vi "数据编码.vi"(0 "table输入":string(combo), 5 "错误常量 2":errorcluster caption="错误输入", 9 "QN":string, 13 "MN":string, 14 "PW":string) -> (4 "错误常量":errorcluster caption="错误输出", 15 "通讯包字符串":string)   [LabVIEW 2016, in "数据传输系统.lvlib"]
panel:
  out "核查数据发送次数":i32
  out "小时数据发送次数":i32
  out "长度":i32
  in  "数据块":T1
  out "通讯包":T2={"包头（2）"="##", "数据段长度（4）"="", "数据段"="", "CRC校验"="", "包尾"=""}
  # "范例代码：\n\n##0101QN=20160801085857223;ST=32;CN=1062;PW=100000;MN=010000A8900016F000169DC0;Flag=5\n;CP=&&RtdInterval=30&&1C80\\r\\n"
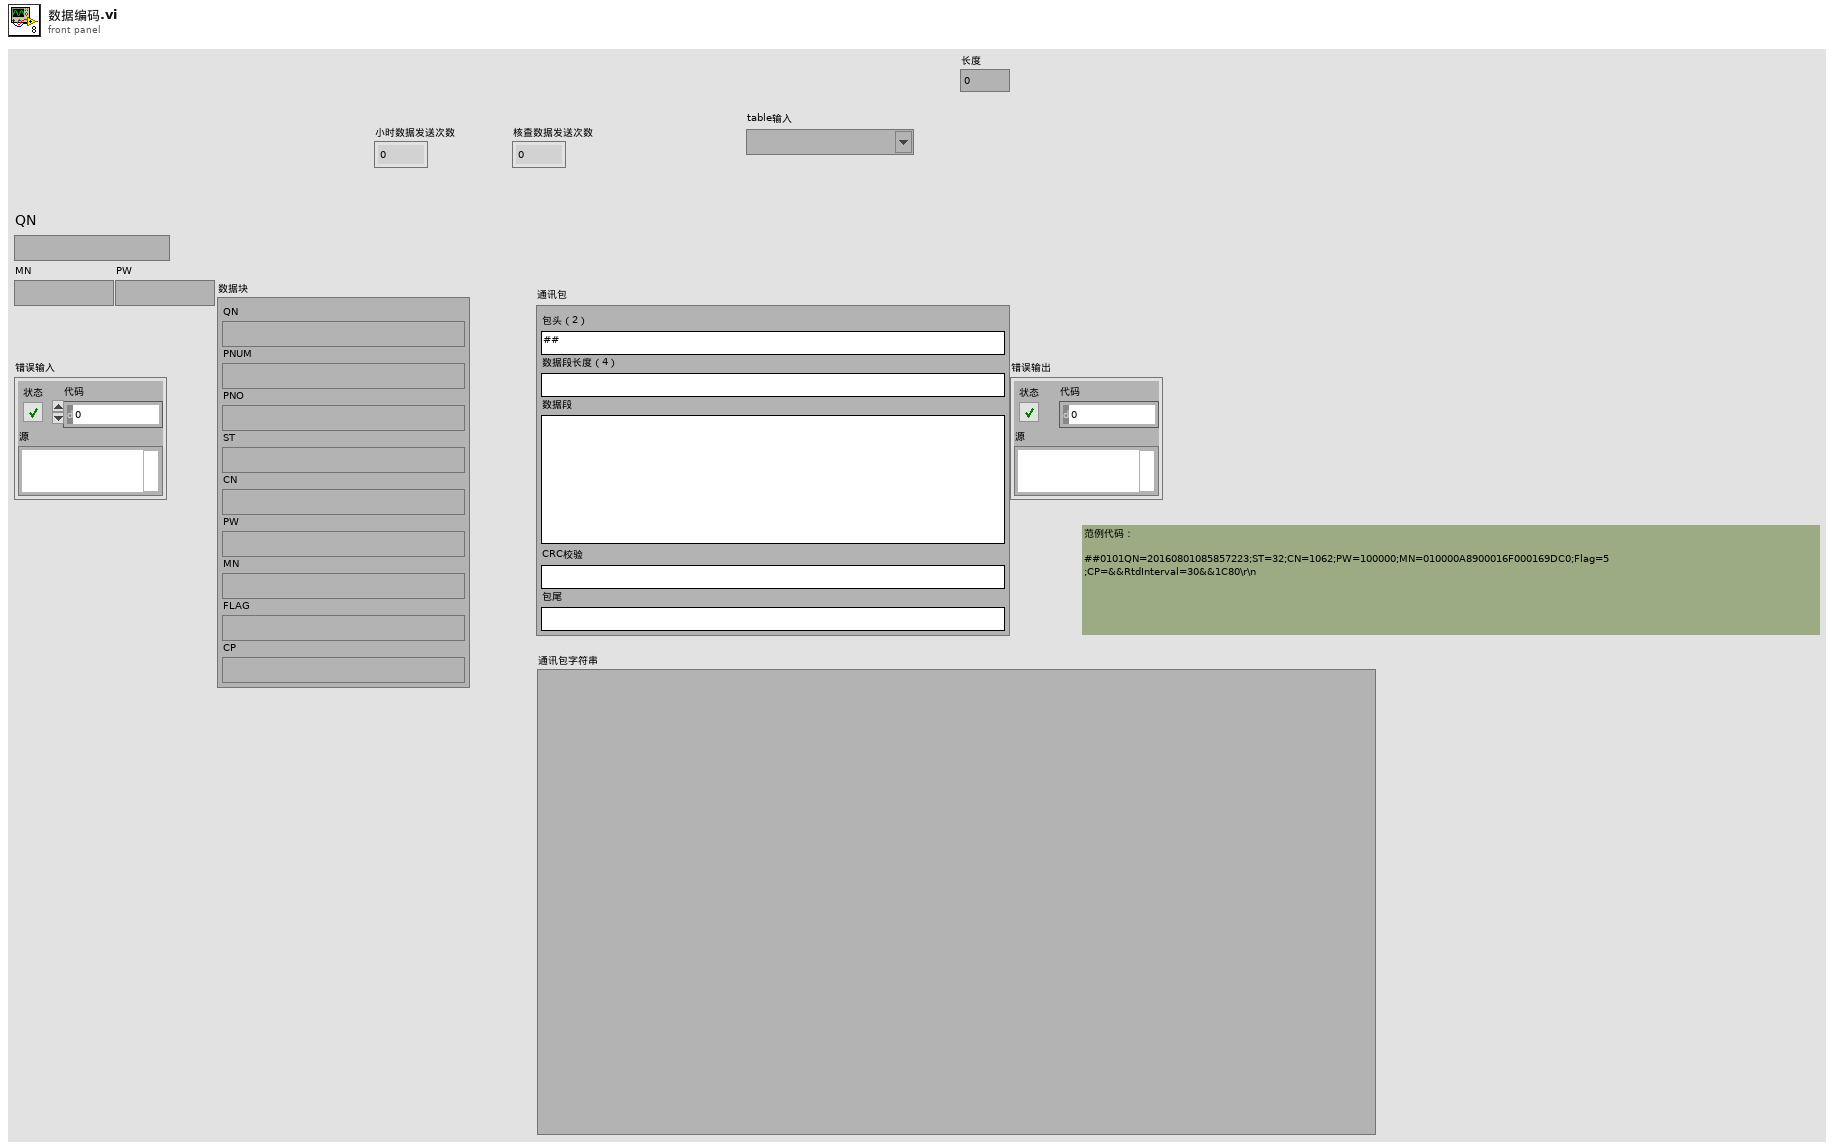
[diagram p1: front panel]
types:
  T1 = cluster{"QN":string, "ST":string, "CN":string, "PW":string, "MN":string, "FLAG":string, "PNUM":string, "PNO":string, "CP":string}
  T2 = cluster{"包头（2）":string, "数据段长度（4）":string, "数据段":string, "CRC校验":string, "包尾":string}
  T3 = cluster{"PH":string[][], "CODCr":string[][], "氨氮":string[][], "CODMn":string[][], "总氮":string[][], "总磷":string[][], "电导率":string[][], "水温":string[][], "DO":string[][], "浊度":string[][], "叶绿素":string[][], "藻密度":string[][], "铜":string[][], "盐度":string[][], "水位":string[][], "流速":string[][], "瞬时流量":string[][], "累积流量":string[][], "亚硝酸盐":string[][], "硫化物":string[][], "ORP":string[][], "铅":string[][], "镉":string[][], "锌":string[][], "镍":string[][], "锰":string[][], "汞":string[][], "气温":string[][], "气压":string[][], "风速":string[][], "风向":string[][]}
  T4 = enum16{"小时数据", "实时数据", "平行样测试", "集成干预测试", "加标回收测试", "核查数据", "空白零点跨度数据", "提取小时数据", "提取实时数据"}
  T5 = enum16{"小时数据", "实时数据", "平行样测试", "集成干预测试", "加标回收测试", "核查数据", "空白零点跨度数据", "提取小时数据", "提取实时数据", "操作日志"}
  T6 = enum16{"小时数据", "实时数据", "平行样测试", "集成干预测试", "加标回收测试", "核查数据", "空白零点跨度数据", "提取小时数据", "提取实时数据", "操作日志", "仪器参数", "3090仪器参数", "提取仪器参数", "报警信息"}
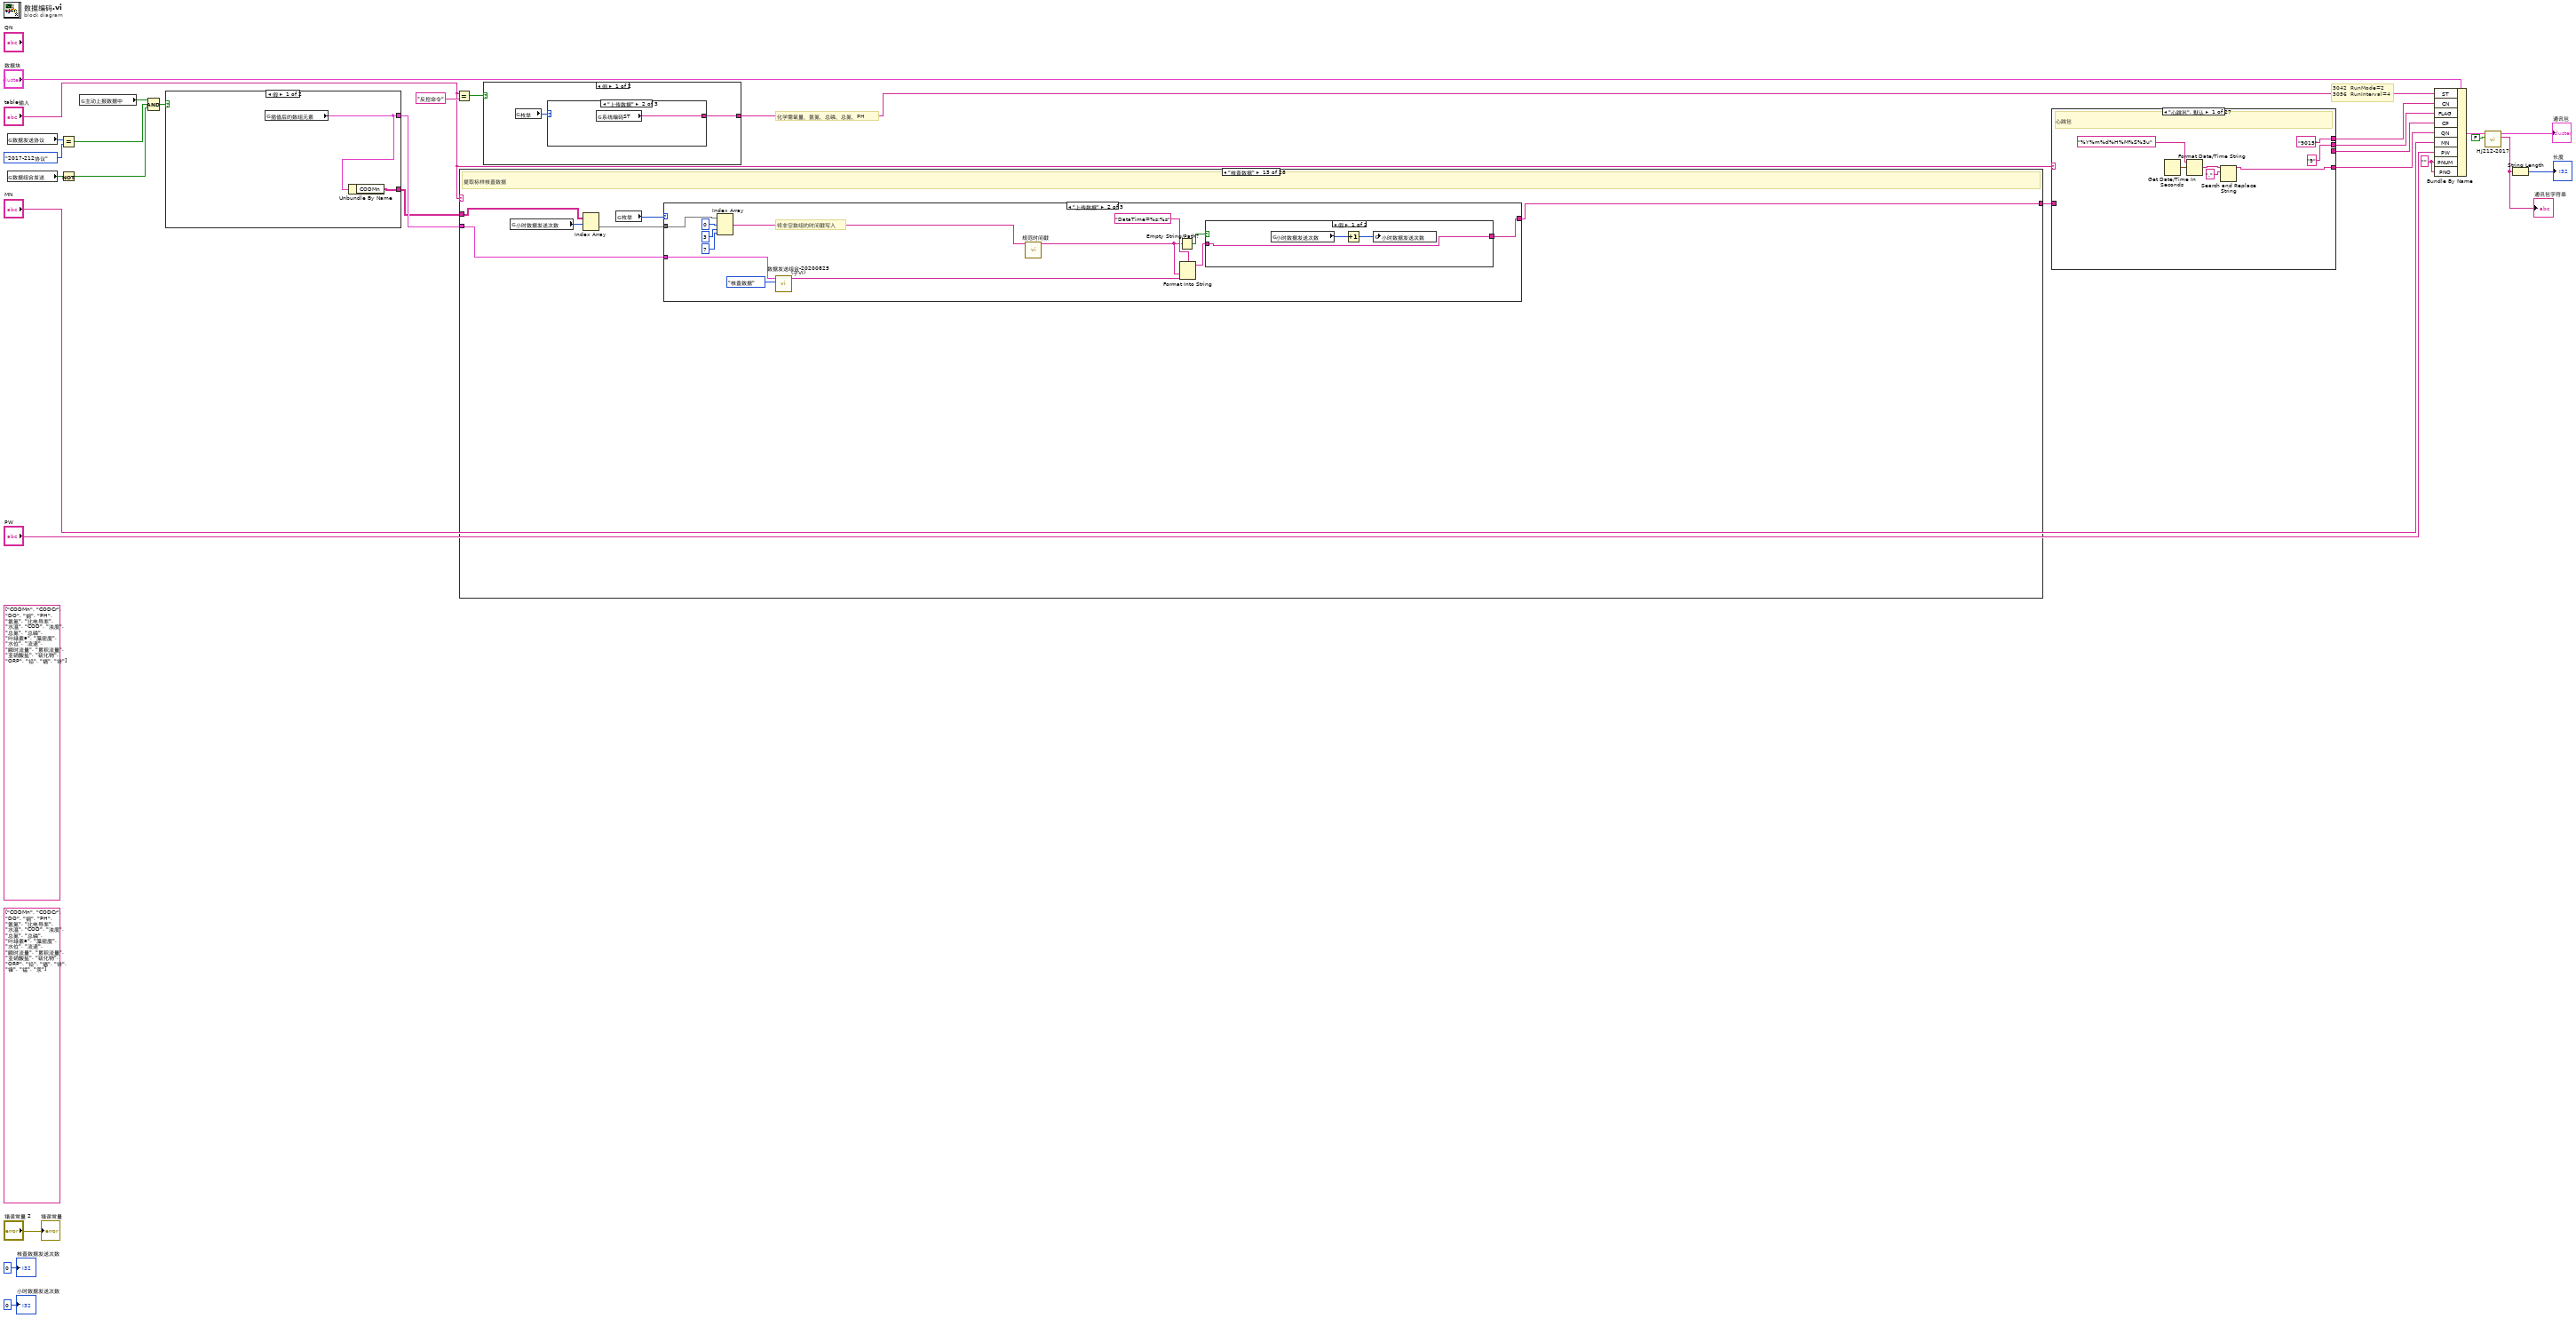
[diagram p0: block diagram]
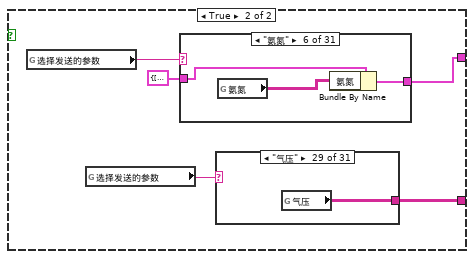
[diagram p2: hidden frame]
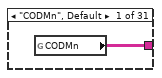
[diagram p3: hidden frame]
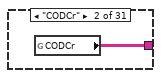
[diagram p4: hidden frame]
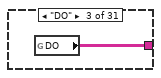
[diagram p5: hidden frame]
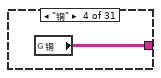
[diagram p6: hidden frame]
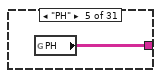
[diagram p7: hidden frame]
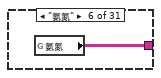
[diagram p8: hidden frame]
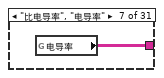
[diagram p9: hidden frame]
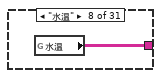
[diagram p10: hidden frame]
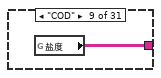
[diagram p11: hidden frame]
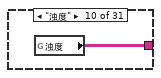
[diagram p12: hidden frame]
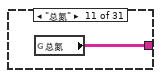
[diagram p13: hidden frame]
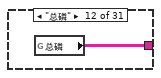
[diagram p14: hidden frame]
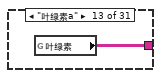
[diagram p15: hidden frame]
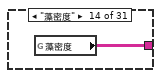
[diagram p16: hidden frame]
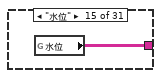
[diagram p17: hidden frame]
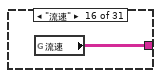
[diagram p18: hidden frame]
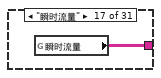
[diagram p19: hidden frame]
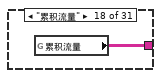
[diagram p20: hidden frame]
diagram:
  (unwired) string[] ["CODMn", "CODCr", "DO", "铜", "PH", "氨氮", "比电导率", "水温", "COD", "浊度", "总氮", "总磷", "叶绿素a", "藻密度", "水位", "流速", "瞬时流量", "累积流量", "亚硝酸盐", "硫化物", "ORP", "铅", "镉", "锌"] ("数组")
  (unwired) string[] ["CODMn", "CODCr", "DO", "铜", "PH", "氨氮", "比电导率", "水温", "COD", "浊度", "总氮", "总磷", "叶绿素a", "藻密度", "水位", "流速", "瞬时流量", "累积流量", "亚硝酸盐", "硫化物", "ORP", "铅", "镉", "锌", "镍", "锰", "汞"] ("数组")
  w15 = ""
  # "化学需氧量、氨氮、总磷、总氮、PH"
  # "3042  RunMode=2\n3056  RunInterval=4"
  n1 = global read "断电保存全局.vi" "数据发送协议"() -> (w5:enum16{"2005-212协议", "2017-212协议"})
  n2 = global read "断电保存全局.vi" "数据组合发送"() -> (w7:bool)
  n3 = Equal?(x=w5, y=enum16{"2005-212协议", "2017-212协议"}."2017-212协议" ("数据发送版本")) -> (x = y?=w8:bool)
  n4 = Not(x=w7) -> (.not. x?=w6:bool)
  n5 = global read "全局 数据发送重叠.vi" "主动上报数据中"() -> (w12:bool)
  n6 = Compound Arithmetic op=AND ("复合运算")(w12, w8, w6) -> (w9:bool)
  n7 = case shown="假" w9 {
    tunnel: [w32 w36] -> w3
    tunnel: [w31 w33] -> w1
    frame False {
      n8 = global read "插值后的新数组.vi" "插值后的数组元素"() -> (w32:T3)
      n9 = Unbundle By Name(w32) -> ("CODMn"=w31:string[][])
    }
    frame True {
      n10 = global read "全局 水样时间.vi" "选择发送的参数"() -> (w37:string)
      n11 = global read "全局 水样时间.vi" "选择发送的参数"() -> (w34:string)
      n12 = case shown="\"氨氮\"" w37 {
        tunnel: T3 {"PH"=[], "CODCr"=[], "氨氮"=[], "CODMn"=[], "总氮"=[], "总磷"=[], "电导率"=[], "水温"=[], "DO"=[], "浊度"=[], "叶绿素"=[], "藻密度"=[], "铜"=[], "盐度"=[], "水位"=[], "流速"=[], "瞬时流量"=[], "累积流量"=[], "亚硝酸盐"=[], "硫化物"=[], "ORP"=[], "铅"=[], "镉"=[], "锌"=[], "镍"=[], "锰"=[], "汞"=[], "气温"=[], "气压"=[], "风速"=[], "风向"=[]} ("插值后的数组元素") -> [w70 w74 w77 w80 w83 w86 w89 w92 w95 w98 w101 w104 w107 w109 w113 w116 w118 w121 w124 w127 w130 w133 w136 w139 w142 w145 w148 w151 w154 w157 w160]
        tunnel: [w69 w72 w75 w78 w81 w84 w88 w91 w93 w96 w99 w102 w105 w108 w111 w114 w117 w120 w123 w126 w129 w132 w135 w138 w141 w144 w147 w150 w153 w156 w159] -> w36
        frame "CODMn", Default {
          n13 = global read "全局 所有参数.vi" "CODMn"() -> (w71:string[][])
          n14 = Bundle By Name(cluster=w70, "CODMn"=w71) -> (w69:T3)
        }
        frame "CODCr" {
          n15 = global read "全局 所有参数.vi" "CODCr"() -> (w73:string[][])
          n16 = Bundle By Name(cluster=w74, "CODCr"=w73) -> (w72:T3)
        }
        frame "DO" {
          n17 = global read "全局 所有参数.vi" "DO"() -> (w76:string[][])
          n18 = Bundle By Name(cluster=w77, "DO"=w76) -> (w75:T3)
        }
        frame "铜" {
          n19 = global read "全局 所有参数.vi" "铜"() -> (w79:string[][])
          n20 = Bundle By Name(cluster=w80, "铜"=w79) -> (w78:T3)
        }
        frame "PH" {
          n21 = global read "全局 所有参数.vi" "PH"() -> (w82:string[][])
          n22 = Bundle By Name(cluster=w83, "PH"=w82) -> (w81:T3)
        }
        frame "氨氮" {
          n23 = global read "全局 所有参数.vi" "氨氮"() -> (w85:string[][])
          n24 = Bundle By Name(cluster=w86, "氨氮"=w85) -> (w84:T3)
        }
        frame "比电导率", "电导率" {
          n25 = global read "全局 所有参数.vi" "电导率"() -> (w87:string[][])
          n26 = Bundle By Name(cluster=w89, "电导率"=w87) -> (w88:T3)
        }
        frame "水温" {
          n27 = global read "全局 所有参数.vi" "水温"() -> (w90:string[][])
          n28 = Bundle By Name(cluster=w92, "水温"=w90) -> (w91:T3)
        }
        frame "COD" {
          n29 = global read "全局 所有参数.vi" "盐度"() -> (w94:string[][])
          n30 = Bundle By Name(cluster=w95, "盐度"=w94) -> (w93:T3)
        }
        frame "浊度" {
          n31 = global read "全局 所有参数.vi" "浊度"() -> (w97:string[][])
          n32 = Bundle By Name(cluster=w98, "浊度"=w97) -> (w96:T3)
        }
        frame "总氮" {
          n33 = global read "全局 所有参数.vi" "总氮"() -> (w100:string[][])
          n34 = Bundle By Name(cluster=w101, "总氮"=w100) -> (w99:T3)
        }
        frame "总磷" {
          n35 = global read "全局 所有参数.vi" "总磷"() -> (w103:string[][])
          n36 = Bundle By Name(cluster=w104, "总磷"=w103) -> (w102:T3)
        }
        frame "叶绿素a" {
          n37 = global read "全局 所有参数.vi" "叶绿素"() -> (w106:string[][])
          n38 = Bundle By Name(cluster=w107, "叶绿素"=w106) -> (w105:T3)
        }
        frame "藻密度" {
          n39 = global read "全局 所有参数.vi" "藻密度"() -> (w110:string[][])
          n40 = Bundle By Name(cluster=w109, "藻密度"=w110) -> (w108:T3)
        }
        frame "水位" {
          n41 = global read "全局 所有参数.vi" "水位"() -> (w112:string[][])
          n42 = Bundle By Name(cluster=w113, "水位"=w112) -> (w111:T3)
        }
        frame "流速" {
          n43 = global read "全局 所有参数.vi" "流速"() -> (w115:string[][])
          n44 = Bundle By Name(cluster=w116, "流速"=w115) -> (w114:T3)
        }
        frame "瞬时流量" {
          n45 = global read "全局 所有参数.vi" "瞬时流量"() -> (w119:string[][])
          n46 = Bundle By Name(cluster=w118, "瞬时流量"=w119) -> (w117:T3)
        }
        frame "累积流量" {
          n47 = global read "全局 所有参数.vi" "累积流量"() -> (w122:string[][])
          n48 = Bundle By Name(cluster=w121, "累积流量"=w122) -> (w120:T3)
        }
        frame "亚硝氮" {
          n49 = global read "全局 所有参数.vi" "亚硝酸盐"() -> (w125:string[][])
          n50 = Bundle By Name(cluster=w124, "亚硝酸盐"=w125) -> (w123:T3)
        }
        frame "硫化物" {
          n51 = global read "全局 所有参数.vi" "硫化物"() -> (w128:string[][])
          n52 = Bundle By Name(cluster=w127, "硫化物"=w128) -> (w126:T3)
        }
        frame "ORP" {
          n53 = global read "全局 所有参数.vi" "ORP"() -> (w131:string[][])
          n54 = Bundle By Name(cluster=w130, "ORP"=w131) -> (w129:T3)
        }
        frame "铅" {
          n55 = global read "全局 所有参数.vi" "铅"() -> (w134:string[][])
          n56 = Bundle By Name(cluster=w133, "铅"=w134) -> (w132:T3)
        }
        frame "镉" {
          n57 = global read "全局 所有参数.vi" "镉"() -> (w137:string[][])
          n58 = Bundle By Name(cluster=w136, "镉"=w137) -> (w135:T3)
        }
        frame "锌" {
          n59 = global read "全局 所有参数.vi" "锌"() -> (w140:string[][])
          n60 = Bundle By Name(cluster=w139, "锌"=w140) -> (w138:T3)
        }
        frame "镍" {
          n61 = global read "全局 所有参数.vi" "镍"() -> (w143:string[][])
          n62 = Bundle By Name(cluster=w142, "镍"=w143) -> (w141:T3)
        }
        frame "锰" {
          n63 = global read "全局 所有参数.vi" "锰"() -> (w146:string[][])
          n64 = Bundle By Name(cluster=w145, "锰"=w146) -> (w144:T3)
        }
        frame "汞" {
          n65 = global read "全局 所有参数.vi" "汞"() -> (w149:string[][])
          n66 = Bundle By Name(cluster=w148, "汞"=w149) -> (w147:T3)
        }
        frame "气温" {
          n67 = global read "全局 所有参数.vi" "气温"() -> (w152:string[][])
          n68 = Bundle By Name(cluster=w151, "气温"=w152) -> (w150:T3)
        }
        frame "气压" {
          n69 = global read "全局 所有参数.vi" "气压"() -> (w155:string[][])
          n70 = Bundle By Name(cluster=w154, "气压"=w155) -> (w153:T3)
        }
        frame "风速" {
          n71 = global read "全局 所有参数.vi" "风速"() -> (w158:string[][])
          n72 = Bundle By Name(cluster=w157, "风速"=w158) -> (w156:T3)
        }
        frame "风向" {
          n73 = global read "全局 所有参数.vi" "风向"() -> (w161:string[][])
          n74 = Bundle By Name(cluster=w160, "风向"=w161) -> (w159:T3)
        }
      }
      n75 = case shown="\"气压\"" w34 {
        tunnel: [w38 w39 w40 w41 w42 w43 w44 w45 w46 w47 w48 w49 w50 w51 w52 w53 w54 w55 w56 w57 w58 w59 w60 w61 w62 w63 w64 w65 w66 w67 w68] -> w33
        frame "CODMn", Default {
          n76 = global read "全局 所有参数.vi" "CODMn"() -> (w38:string[][])
        }
        frame "CODCr" {
          n77 = global read "全局 所有参数.vi" "CODCr"() -> (w39:string[][])
        }
        frame "DO" {
          n78 = global read "全局 所有参数.vi" "DO"() -> (w40:string[][])
        }
        frame "铜" {
          n79 = global read "全局 所有参数.vi" "铜"() -> (w41:string[][])
        }
        frame "PH" {
          n80 = global read "全局 所有参数.vi" "PH"() -> (w42:string[][])
        }
        frame "氨氮" {
          n81 = global read "全局 所有参数.vi" "氨氮"() -> (w43:string[][])
        }
        frame "比电导率", "电导率" {
          n82 = global read "全局 所有参数.vi" "电导率"() -> (w44:string[][])
        }
        frame "水温" {
          n83 = global read "全局 所有参数.vi" "水温"() -> (w45:string[][])
        }
        frame "COD" {
          n84 = global read "全局 所有参数.vi" "盐度"() -> (w46:string[][])
        }
        frame "浊度" {
          n85 = global read "全局 所有参数.vi" "浊度"() -> (w47:string[][])
        }
        frame "总氮" {
          n86 = global read "全局 所有参数.vi" "总氮"() -> (w48:string[][])
        }
        frame "总磷" {
          n87 = global read "全局 所有参数.vi" "总磷"() -> (w49:string[][])
        }
        frame "叶绿素a" {
          n88 = global read "全局 所有参数.vi" "叶绿素"() -> (w50:string[][])
        }
        frame "藻密度" {
          n89 = global read "全局 所有参数.vi" "藻密度"() -> (w51:string[][])
        }
        frame "水位" {
          n90 = global read "全局 所有参数.vi" "水位"() -> (w52:string[][])
        }
        frame "流速" {
          n91 = global read "全局 所有参数.vi" "流速"() -> (w53:string[][])
        }
        frame "瞬时流量" {
          n92 = global read "全局 所有参数.vi" "瞬时流量"() -> (w54:string[][])
        }
        frame "累积流量" {
          n93 = global read "全局 所有参数.vi" "累积流量"() -> (w55:string[][])
        }
        frame "亚硝氮" {
          n94 = global read "全局 所有参数.vi" "亚硝酸盐"() -> (w56:string[][])
        }
        frame "硫化物" {
          n95 = global read "全局 所有参数.vi" "硫化物"() -> (w57:string[][])
        }
        frame "ORP" {
          n96 = global read "全局 所有参数.vi" "ORP"() -> (w58:string[][])
        }
        frame "铅" {
          n97 = global read "全局 所有参数.vi" "铅"() -> (w59:string[][])
        }
        frame "镉" {
          n98 = global read "全局 所有参数.vi" "镉"() -> (w60:string[][])
        }
        frame "锌" {
          n99 = global read "全局 所有参数.vi" "锌"() -> (w61:string[][])
        }
        frame "镍" {
          n100 = global read "全局 所有参数.vi" "镍"() -> (w62:string[][])
        }
        frame "锰" {
          n101 = global read "全局 所有参数.vi" "锰"() -> (w63:string[][])
        }
        frame "汞" {
          n102 = global read "全局 所有参数.vi" "汞"() -> (w64:string[][])
        }
        frame "气温" {
          n103 = global read "全局 所有参数.vi" "气温"() -> (w65:string[][])
        }
        frame "气压" {
          n104 = global read "全局 所有参数.vi" "气压"() -> (w66:string[][])
        }
        frame "风速" {
          n105 = global read "全局 所有参数.vi" "风速"() -> (w67:string[][])
        }
        frame "风向" {
          n106 = global read "全局 所有参数.vi" "风向"() -> (w68:string[][])
        }
      }
    }
  }
  n107 = Equal?(x="table输入", y="反控命令") -> (x = y?=w19:bool)
  n108 = case shown="\"核查数据\"" "table输入" {
    tunnel: [w163 w170 w184 w227 w250 _ w264 w273 w284 w434 w465 w512 w563 w592 w624 w655 w681 w710 w739 w776 w810 w841 w869 w892 w925 w948 w959 w970] -> w13
    tunnel: w1 -> [_ _ _ _ _ _ _ _ w281 w433 _ _ w562 w593 w619 w650 w682 w709 w738 w775 w809 w840 _ w891 _ _ _ _]
    tunnel: w3 -> [_ _ _ _ _ _ _ _ w282 w435 _ _ w558 w588 w620 w651 w680 w708 w737 w771 w805 w836 w867 w887 _ _ _ _]
    frame "反控命令" {
      n109 = global read "全局 反控命令枚举.vi" "反控命令枚举"() -> (w162:enum16{"返回请求应答", "返回执行结果"})
      n110 = case shown="\"返回执行结果\"" w162 {
        tunnel: ["QnRtn=1" w166] -> w163
        frame "返回请求应答", Default {
        }
        frame "返回执行结果" {
          n111 = global read "全局 反控命令枚举.vi" "执行结果定义"() -> (w167:u16)
          n112 = Number To Decimal String(number=w167) -> (decimal integer string=w165:string)  [unwired: 1 in]
          n113 = Concatenate Strings("ExeRtn=", w165) -> (w166:string)
        }
      }
    }
    frame "超标留样返回" {
      n114 = global read "全局1.vi" "枚举"() -> (w169:enum16{"返回请求应答", "上传数据", "返回执行结果"})
      n115 = case shown="\"返回请求应答\", 默认" w169 {
        tunnel: ["QnRtn=1" w172 "ExeRtn=1"] -> w170
        frame "返回请求应答", Default {
        }
        frame "上传数据" {
          n116 = global read "全局1.vi" "register values"() -> (w181:u16[])
          n117 = Get Date/Time In Seconds() -> (seconds since 1Jan1904=w179:timestamp)
          n118 = Index Array(array=w181, index=7 ("索引")) -> (element=w174:u16)
          n119 = Format Date/Time String(time format string (%c)="%Y%m%d%H%M%S" ("时间格式字符串(%c)"), seconds (now)=w179) -> (date/time string=w177:string)  [unwired: 1 in]
          n120 = Number To Decimal String(number=w174) -> (decimal integer string=w175:string)  [unwired: 1 in]
          n121 = Format Into String(format string="VaseNo=%s" ("格式字符串"), w175) -> (resulting string=w173:string)  [unwired: 2 in, 1 out]
          n122 = Format Into String(format string="DataTime=%s;%s" ("格式字符串"), w177, w173) -> (resulting string=w172:string)  [unwired: 2 in, 1 out]
        }
        frame "返回执行结果" {
        }
      }
    }
    frame "提取经纬度环境信息" {
      # "BDS纬度"
      # "BDS纬度"
      # "GPS纬度"
      # "GPS经度"
      # "湿度"
      # "温度"
      # "电压"
      # "时间"
      n123 = global read "全局1.vi" "枚举"() -> (w185:enum16{"返回请求应答", "上传数据", "返回执行结果"})
      n124 = case shown="\"上传数据\"" w185 {
        tunnel: ["QnRtn=1" w198 "ExeRtn=1"] -> w184
        frame "返回请求应答", Default {
        }
        frame "上传数据" {
          n125 = global read "全局 环境参数.vi" "环境参数"() -> (w188:string[][])
          n126 = global read "全局 环境参数.vi" "columns输出"() -> (w195:string[])
          n127 = Index Array(array=w188, index (row)=0 ("索引 (行)")) -> (element=w191:string[])  [unwired: 1 in]
          n128 = Get Date/Time In Seconds() -> (seconds since 1Jan1904=w200:timestamp)
          n129 = Array Subset(array=w195, index=1 ("索引")) -> (w196:string[])  [unwired: 1 in]
          n130 = for {
            tunnel: w196 -> [w204] mode=indexing
            tunnel: [w203] -> w197 mode=indexing
            n131 = case shown="\"BDS经度\"" w204 {
              tunnel: ["" "Volt=%s;" "Temp=%s;" ("格式字符串") "Hum=%s;" ("格式字符串") "Lng=%s;" "Lat=%s;" "Lng2=%s;" "Lat2=%s;"] -> w203
              frame "假", Default {
              }
              frame "电压" {
              }
              frame "室温" {
              }
              frame "湿度" {
              }
              frame "GPS经度" {
              }
              frame "GPS纬度" {
              }
              frame "BDS经度" {
              }
              frame "BDS纬度" {
              }
            }
          }
          n132 = Format Date/Time String(time format string (%c)="%Y%m%d%H%M%S" ("时间格式字符串(%c)"), seconds (now)=w200) -> (date/time string=w199:string)  [unwired: 1 in]
          n133 = Array Subset(array=w191, index=1 ("索引")) -> (w193:string[])  [unwired: 1 in]
          n134 = for {
            shift-right: [w218] -> w187
            shift-left: "" -> [w217]
            tunnel: w197 -> [w216] mode=indexing
            tunnel: w193 -> [w214] mode=indexing
            n135 = Empty String/Path?(string/path=w214) -> (empty?=w220:bool)
            n136 = Fract/Exp String To Number(string=w214) -> (number=w215:dbl)  [unwired: 3 in, 1 out]
            n137 = Number To Fractional String(number=w215) -> (F-format string=w213:string)  [unwired: 3 in]
            n138 = case shown="假" w220 {
              tunnel: [w223 w224] -> w219
              tunnel: w216 -> [w222 _]
              tunnel: w213 -> [w221 _]
              tunnel: w213 -> [_ w224]
              frame False {
                n139 = Format Into String(format string=w222, w221) -> (resulting string=w223:string)  [unwired: 2 in, 1 out]
              }
              frame True {
              }
            }
            n140 = Concatenate Strings(w217, w219) -> (w218:string)
          }
          n141 = Format Into String(format string="DataTime=%s;%s" ("格式字符串"), w199, w187) -> (resulting string=w198:string)  [unwired: 2 in, 1 out]
        }
        frame "返回执行结果" {
        }
      }
    }
    frame "提取现场系统信息" {
      n142 = global read "全局1.vi" "枚举"() -> (w226:enum16{"返回请求应答", "上传数据", "返回执行结果"})
      n143 = case shown="\"上传数据\"" w226 {
        tunnel: ["QnRtn=1" w247 "ExeRtn=1"] -> w227
        frame "返回请求应答", Default {
        }
        frame "上传数据" {
          n144 = global read "全局1.vi" "register values"() -> (w246:u16[])
          n145 = Index Array(array=w246, index #1=0 ("索引"), index #2=6 ("索引")) -> (element #1=w242:u16, element #2=w229:u16)
          n146 = Number To Decimal String(number=w242) -> (decimal integer string=w244:string)  [unwired: 1 in]
          n147 = Number To Decimal String(number=w229) -> (decimal integer string=w238:string)  [unwired: 1 in]
          n148 = Get Date/Time In Seconds() -> (seconds since 1Jan1904=w232:timestamp)
          n149 = Format Date/Time String(time format string (%c)="%Y%m%d%H%M%S%u" ("时间格式字符串(%c)"), seconds (now)=w232) -> (date/time string=w235:string)  [unwired: 1 in]
          n150 = Format Into String(format string="RunMode=%s;" ("格式字符串"), w244) -> (resulting string=w241:string)  [unwired: 2 in, 1 out]
          n151 = Format Into String(format string="RunInterval=%s;" ("格式字符串"), w238) -> (resulting string=w239:string)  [unwired: 2 in, 1 out]
          n152 = Search and Replace String(input string=w235, search string="." ("搜索字符串")) -> (result string=w231:string)  [unwired: 6 in, 3 out]
          n153 = Format Into String(format string="SystemTime=%s;" ("格式字符串"), w231) -> (resulting string=w236:string)  [unwired: 2 in, 1 out]
          n154 = Concatenate Strings(w241, w239, w236) -> (w247:string)
        }
        frame "返回执行结果" {
        }
      }
    }
    frame "提取监测仪表时间" {
      n155 = global read "全局1.vi" "枚举"() -> (w249:enum16{"返回请求应答", "上传数据", "返回执行结果"})
      n156 = case shown="\"上传数据\"" w249 {
        tunnel: ["QnRtn=1" w262 "ExeRtn=1"] -> w250
        frame "返回请求应答", Default {
        }
        frame "上传数据" {
          n157 = global read "全局 提取仪器参数.vi" "仪器编码"() -> (w252:string)
          n158 = Format Into String(format string="PolId=%s;" ("格式字符串"), w252) -> (resulting string=w260:string)  [unwired: 2 in, 1 out]
          n159 = Get Date/Time In Seconds() -> (seconds since 1Jan1904=w255:timestamp)
          n160 = Format Date/Time String(time format string (%c)="%Y%m%d%H%M%S%u" ("时间格式字符串(%c)"), seconds (now)=w255) -> (date/time string=w258:string)  [unwired: 1 in]
          n161 = Search and Replace String(input string=w258, search string="." ("搜索字符串")) -> (result string=w254:string)  [unwired: 6 in, 3 out]
          n162 = Format Into String(format string="SystemTime=%s;" ("格式字符串"), w254) -> (resulting string=w253:string)  [unwired: 2 in, 1 out]
          n163 = Concatenate Strings(w260, w253) -> (w262:string)
        }
        frame "返回执行结果" {
        }
      }
    }
    frame "心跳包", Default {
    }
    frame "提取数采仪时间" {
      (unwired) ""
      n164 = global read "全局1.vi" "枚举"() -> (w265:enum16{"返回请求应答", "上传数据", "返回执行结果"})
      n165 = case shown="\"上传数据\"" w265 {
        tunnel: ["QnRtn=1" w267 "ExeRtn=1"] -> w264
        frame "返回请求应答", Default {
        }
        frame "上传数据" {
          n166 = Get Date/Time In Seconds() -> (seconds since 1Jan1904=w271:timestamp)
          n167 = Format Date/Time String(time format string (%c)="%Y%m%d%H%M%S" ("时间格式字符串(%c)"), seconds (now)=w271) -> (date/time string=w268:string)  [unwired: 1 in]
          n168 = Concatenate Strings("SystemTime=", w268) -> (w267:string)
        }
        frame "返回执行结果" {
        }
      }
    }
    frame "提取实时数据间隔" {
      (unwired) ""
      n169 = global read "全局1.vi" "枚举"() -> (w274:enum16{"返回请求应答", "上传数据", "返回执行结果"})
      n170 = case shown="\"上传数据\"" w274 {
        tunnel: ["QnRtn=1" w278 "ExeRtn=1"] -> w273
        frame "返回请求应答", Default {
        }
        frame "上传数据" {
          n171 = global read "实时数据发送间隔全局.vi" "实时数据发送间隔"() -> (w277:u32)
          n172 = Number To Decimal String(number=w277) -> (decimal integer string=w276:string)  [unwired: 1 in]
          n173 = Concatenate Strings("RtdInterval=", w276) -> (w278:string)
        }
        frame "返回执行结果" {
        }
      }
    }
    frame "实时数据" {
      # "包含质控数据主动上传"
      n174 = global read "全局 实时数据参数.vi" "实时数据参数"() -> (w283:string)
      n175 = case shown="\"水样测试\", 默认" w283 {
        tunnel: [w287 w312 w337 w368 w392 w413] -> w284
        tunnel: w282 -> [w286 w311 w336 w366 w390 w411]
        tunnel: w281 -> [w285 w310 w335 w365 w389 w410]
        frame "水样测试", Default {
          n176 = global read "全局1.vi" "枚举"() -> (w288:enum16{"返回请求应答", "上传数据", "返回执行结果"})
          n177 = case shown="\"上传数据\"" w288 {
            tunnel: ["QnRtn=1" w306 "ExeRtn=1"] -> w287
            tunnel: w286 -> [_ w292 _]
            tunnel: w285 -> [_ w290 _]
            frame "返回请求应答", Default {
            }
            frame "上传数据" {
              n178 = call "数据发送组合-20200825 (子VI).vi"("枚举"=T4."实时数据", "插值后的数组元素"=w292) -> ("字符串"=w293:string)  [unwired: 9 in]
              n179 = global read "全局 小时数据发送次数.vi" "小时数据发送次数"() -> (w304:i32)
              n180 = Empty String/Path?(string/path=w293) -> (empty?=w305:bool)
              n181 = Index Array(array=w290, index (row)=w304) -> (element=w303:string[])  [unwired: 1 in]
              n182 = Index Array(array=w303, index=0 ("索引")) -> (element=w301:string)
              n183 = call "规范时间戳.vi"("字符串"=w301) -> ("result string"=w299:string)  [unwired: 10 in]
              n184 = Format Into String(format string="DataTime=%s;", w299) -> (resulting string=w298:string)  [unwired: 2 in, 1 out]
              n185 = Concatenate Strings(w298, w293) -> (w295:string)
              n186 = String Length(string=w295) -> (length=w297:i32)
              n187 = Decrement(x=w297) -> (x-1=w296:i32)
              n188 = String Subset(string=w295, length (rest)=w296) -> (substring=w294:string)  [unwired: 1 in]
              n189 = case shown="假" w305 {
                tunnel: [w307 ""] -> w306
                tunnel: w294 -> [w307 _]
                frame False {
                }
                frame True {
                }
              }
            }
            frame "返回执行结果" {
            }
          }
        }
        frame "平行样测试" {
          n190 = global read "全局1.vi" "枚举"() -> (w313:enum16{"返回请求应答", "上传数据", "返回执行结果"})
          n191 = case shown="\"上传数据\"" w313 {
            tunnel: ["QnRtn=1" w325 "ExeRtn=1"] -> w312
            tunnel: w310 -> [_ w319 _]
            tunnel: w311 -> [_ w316 _]
            frame "返回请求应答", Default {
            }
            frame "上传数据" {
              # "CODMn"
              n192 = call "数据发送组合-20200825 (子VI).vi"("枚举"=T4."平行样测试", "插值后的数组元素"=w316) -> ("字符串"=w315:string)  [unwired: 9 in]
              n193 = global read "全局 小时数据发送次数.vi" "小时数据发送次数"() -> (w318:i32)
              n194 = Index Array(array=w319, index (row)=w318) -> (element=w323:string[])  [unwired: 1 in]
              n195 = Index Array(array=w323, index=0 ("索引")) -> (element=w320:string)
              n196 = call "规范时间戳.vi"("字符串"=w320) -> ("result string"=w321:string)  [unwired: 10 in]
              n197 = Empty String/Path?(string/path=w320) -> (empty?=w324:bool)
              n198 = Format Into String(format string="DataTime=%s;%s" ("格式字符串"), w321, w315) -> (resulting string=w326:string)  [unwired: 2 in, 1 out]
              n199 = case shown="真" w324 {
                tunnel: [w330 ""] -> w325
                tunnel: w326 -> [w330 _]
                frame False {
                  n200 = global read "全局 小时数据发送次数.vi" "小时数据发送次数"() -> (w329:i32)
                  n201 = Increment(x=w329) -> (x+1=w328:i32)
                  n202 = global write "全局 小时数据发送次数.vi" "小时数据发送次数"(w328) -> ()
                }
                frame True {
                  n203 = global read "全局 小时数据发送次数.vi" "小时数据发送次数"() -> (w332:i32)
                  n204 = Increment(x=w332) -> (x+1=w331:i32)
                  n205 = global write "全局 小时数据发送次数.vi" "小时数据发送次数"(w331) -> ()
                }
              }
            }
            frame "返回执行结果" {
            }
          }
        }
        frame "集成干预测试" {
          n206 = global read "全局1.vi" "枚举"() -> (w338:enum16{"返回请求应答", "上传数据", "返回执行结果"})
          n207 = case shown="\"上传数据\"" w338 {
            tunnel: ["QnRtn=1" w351 "ExeRtn=1"] -> w337
            tunnel: w335 -> [_ w345 _]
            tunnel: w336 -> [_ w342 _]
            frame "返回请求应答", Default {
            }
            frame "上传数据" {
              # "CODMn"
              n208 = global read "全局 小时数据发送次数.vi" "小时数据发送次数"() -> (w344:i32)
              n209 = call "数据发送组合-20200825 (子VI).vi"("枚举"=T4."集成干预测试", "插值后的数组元素"=w342) -> ("字符串"=w341:string)  [unwired: 9 in]
              n210 = Index Array(array=w345, index (row)=w344) -> (element=w349:string[])  [unwired: 1 in]
              n211 = Index Array(array=w349, index=0 ("索引")) -> (element=w346:string)
              n212 = global read "断电保存全局.vi" "应用环境"() -> (w340:enum16{"STD", "GB212"})
              n213 = case shown="\"STD\", 默认" w340 {
                tunnel: [w355 w356] -> w347
                tunnel: w346 -> [w354 w357]
                frame "STD", Default {
                  n214 = call "规范时间戳.vi"("字符串"=w354) -> ("result string"=w355:string)  [unwired: 10 in]
                }
                frame "GB212" {
                  n215 = call "规范分钟数据时间戳.vi"("字符串"=w357) -> ("result string"=w356:string)  [unwired: 10 in]
                }
              }
              n216 = Empty String/Path?(string/path=w346) -> (empty?=w350:bool)
              n217 = Format Into String(format string="DataTime=%s;%s" ("格式字符串"), w347, w341) -> (resulting string=w352:string)  [unwired: 2 in, 1 out]
              n218 = case shown="假" w350 {
                tunnel: [w360 ""] -> w351
                tunnel: w352 -> [w360 _]
                frame False {
                  n219 = global read "全局 小时数据发送次数.vi" "小时数据发送次数"() -> (w359:i32)
                  n220 = Increment(x=w359) -> (x+1=w358:i32)
                  n221 = global write "全局 小时数据发送次数.vi" "小时数据发送次数"(w358) -> ()
                }
                frame True {
                  n222 = global read "全局 小时数据发送次数.vi" "小时数据发送次数"() -> (w362:i32)
                  n223 = Increment(x=w362) -> (x+1=w361:i32)
                  n224 = global write "全局 小时数据发送次数.vi" "小时数据发送次数"(w361) -> ()
                }
              }
            }
            frame "返回执行结果" {
            }
          }
        }
        frame "加标回收测试" {
          n225 = global read "全局1.vi" "枚举"() -> (w367:enum16{"返回请求应答", "上传数据", "返回执行结果"})
          n226 = case shown="\"上传数据\"" w367 {
            tunnel: ["QnRtn=1" w378 "ExeRtn=1"] -> w368
            tunnel: w365 -> [_ w373 _]
            tunnel: w366 -> [_ w375 _]
            frame "返回请求应答", Default {
            }
            frame "上传数据" {
              # "w01001-Check=63.0,w01001-WaterTime=20160801080000,w01001-Water=45.23,w01001-Chroma=1000,w01001-Volume=0.2,w01001-DVolume=200,w01003-Flag=N;"
              # "CODMn"
              n227 = global read "全局 小时数据发送次数.vi" "小时数据发送次数"() -> (w372:i32)
              n228 = call "加标回收数据组合 (子VI).vi"("小时数据发送次数"=w372, "数据"=w373, "污染物编码"="CODMn") -> ("datatime"=w371:string)  [unwired: 7 in, 1 out]
              n229 = call "规范时间戳.vi"("字符串"=w371) -> ("result string"=w380:string)  [unwired: 10 in]
              n230 = Empty String/Path?(string/path=w380) -> (empty?=w377:bool)
              n231 = call "数据发送组合-20200825 (子VI).vi"("枚举"=T4."加标回收测试", "插值后的数组元素"=w375) -> ("字符串"=w374:string)  [unwired: 9 in]
              n232 = Format Into String(format string="DataTime=%s;%s" ("格式字符串"), w380, w374) -> (resulting string=w379:string)  [unwired: 2 in, 1 out]
              n233 = case shown="真" w377 {
                tunnel: [w384 ""] -> w378
                tunnel: w379 -> [w384 _]
                frame False {
                  n234 = global read "全局 小时数据发送次数.vi" "小时数据发送次数"() -> (w383:i32)
                  n235 = Increment(x=w383) -> (x+1=w382:i32)
                  n236 = global write "全局 小时数据发送次数.vi" "小时数据发送次数"(w382) -> ()
                }
                frame True {
                  n237 = global read "全局 小时数据发送次数.vi" "小时数据发送次数"() -> (w386:i32)
                  n238 = Increment(x=w386) -> (x+1=w385:i32)
                  n239 = global write "全局 小时数据发送次数.vi" "小时数据发送次数"(w385) -> ()
                }
              }
            }
            frame "返回执行结果" {
            }
          }
        }
        frame "核查数据" {
          n240 = global read "全局1.vi" "枚举"() -> (w391:enum16{"返回请求应答", "上传数据", "返回执行结果"})
          n241 = case shown="\"上传数据\"" w391 {
            tunnel: ["QnRtn=1" w402 "ExeRtn=1"] -> w392
            tunnel: w390 -> [_ w395 _]
            tunnel: w389 -> [_ w394 _]
            frame "返回请求应答", Default {
            }
            frame "上传数据" {
              # "将非空数组的时间戳写入"
              n242 = call "数据发送组合-20200825 (子VI).vi"("枚举"=T4."核查数据", "插值后的数组元素"=w395) -> ("字符串"=w396:string)  [unwired: 9 in]
              n243 = global read "全局 小时数据发送次数.vi" "小时数据发送次数"() -> (w398:i32)
              n244 = Index Array(array=w394, index (row)=w398) -> (element=w401:string[])  [unwired: 1 in]
              n245 = Index Array(array=w401, index=0 ("索引")) -> (element=w400:string)
              n246 = call "规范分钟数据时间戳.vi"("字符串"=w400) -> ("result string"=w399:string)  [unwired: 10 in]
              n247 = Empty String/Path?(string/path=w399) -> (empty?=w404:bool)
              n248 = Format Into String(format string="DataTime=%s;%s" ("格式字符串"), w399, w396) -> (resulting string=w403:string)  [unwired: 2 in, 1 out]
              n249 = case shown="假" w404 {
                tunnel: [w407 ""] -> w402
                tunnel: w403 -> [w407 _]
                frame False {
                }
                frame True {
                }
              }
            }
            frame "返回执行结果" {
            }
          }
        }
        frame "空白测试", "跨度核查" {
          n250 = global read "全局1.vi" "枚举"() -> (w412:enum16{"返回请求应答", "上传数据", "返回执行结果"})
          n251 = case shown="\"上传数据\"" w412 {
            tunnel: ["QnRtn=1" w423 "ExeRtn=1"] -> w413
            tunnel: w411 -> [_ w417 _]
            tunnel: w410 -> [_ w415 _]
            frame "返回请求应答", Default {
            }
            frame "上传数据" {
              n252 = global read "全局 小时数据发送次数.vi" "小时数据发送次数"() -> (w421:i32)
              n253 = call "数据发送组合-20200825 (子VI).vi"("枚举"=T4."空白零点跨度数据", "插值后的数组元素"=w417) -> ("字符串"=w416:string)  [unwired: 9 in]
              n254 = Index Array(array=w415, index (row)=w421) -> (element=w427:string[])  [unwired: 1 in]
              n255 = Index Array(array=w427, index #1=0 ("索引"), index #2=3 ("索引"), index #3=7 ("索引")) -> (element #1=w420:string)  [unwired: 2 out]
              n256 = call "规范小时时间戳.vi"("字符串"=w420) -> ("result string"=w419:string)  [unwired: 10 in]
              n257 = Empty String/Path?(string/path=w419) -> (empty?=w424:bool)
              n258 = Format Into String(format string="DataTime=%s;%s" ("格式字符串"), w419, w416) -> (resulting string=w422:string)  [unwired: 2 in, 1 out]
              n259 = case shown="假" w424 {
                tunnel: [w430 ""] -> w423
                tunnel: w422 -> [w430 _]
                frame False {
                }
                frame True {
                }
              }
            }
            frame "返回执行结果" {
            }
          }
        }
      }
    }
    frame "小时数据" {
      # "发送小时数据"
      n260 = global read "全局1.vi" "枚举"() -> (w436:enum16{"返回请求应答", "上传数据", "返回执行结果"})
      n261 = case shown="\"上传数据\"" w436 {
        tunnel: ["QnRtn=1" w458 "ExeRtn=1"] -> w434
        tunnel: w435 -> [_ w446 _]
        tunnel: w433 -> [_ w443 _]
        frame "返回请求应答", Default {
          (unwired) 0 ("当前包数")
          n262 = global read "全局 数据数组大小.vi" "数据数组大小"() -> (w437:i32)
          n263 = global write "全局1.vi" "枚举"(enum16{"返回请求应答", "上传数据", "返回执行结果"}."上传数据" ("枚举")) -> ()
          n264 = Equal To 0?(x=w437) -> (x = 0?=w438:bool)
          n265 = case shown="真" w438 {
            frame False {
            }
            frame True {
              n266 = global read "全局 小时数据发送次数.vi" "小时数据发送次数"() -> (w442:i32)
              n267 = Increment(x=w442) -> (x+1=w441:i32)
              n268 = global write "全局 小时数据发送次数.vi" "小时数据发送次数"(w441) -> ()
            }
          }
        }
        frame "上传数据" {
          n269 = call "数据发送组合-20200825 (子VI).vi"("枚举"=enum16{"小时数据", "实时数据"}."小时数据", "插值后的数组元素"=w446) -> ("字符串"=w444:string)  [unwired: 9 in]
          n270 = global read "全局 小时数据发送次数.vi" "小时数据发送次数"() -> (w457:i32)
          n271 = Empty String/Path?(string/path=w444) -> (empty?=w459:bool)
          n272 = Index Array(array=w443, index (row)=w457) -> (element=w456:string[])  [unwired: 1 in]
          n273 = Index Array(array=w456, index=0 ("索引")) -> (element=w454:string)
          n274 = call "规范小时时间戳.vi"("字符串"=w454) -> ("result string"=w451:string)  [unwired: 10 in]
          n275 = Format Into String(format string="DataTime=%s;", w451) -> (resulting string=w453:string)  [unwired: 2 in, 1 out]
          n276 = Concatenate Strings(w453, w444) -> (w448:string)
          n277 = String Length(string=w448) -> (length=w450:i32)
          n278 = Decrement(x=w450) -> (x-1=w449:i32)
          n279 = String Subset(string=w448, length (rest)=w449) -> (substring=w447:string)  [unwired: 1 in]
          n280 = case shown="假" w459 {
            tunnel: [w460 ""] -> w458
            tunnel: w447 -> [w460 _]
            frame False {
            }
            frame True {
            }
          }
        }
        frame "返回执行结果" {
          (unwired) 0 ("当前包数")
          n281 = global write "全局1.vi" "枚举"(enum16{"返回请求应答", "上传数据", "返回执行结果"}."返回请求应答" ("枚举")) -> ()
        }
      }
    }
    frame "剖面多参数H" {
      # "发送小时数据"
      n282 = global read "全局1.vi" "枚举"() -> (w464:enum16{"返回请求应答", "上传数据", "返回执行结果"})
      n283 = case shown="\"上传数据\"" w464 {
        tunnel: ["QnRtn=1" w474 "ExeRtn=1"] -> w465
        frame "返回请求应答", Default {
          (unwired) 0 ("当前包数")
          n284 = global read "全局 数据数组大小.vi" "数据数组大小"() -> (w466:i32)
          n285 = global write "全局1.vi" "枚举"(enum16{"返回请求应答", "上传数据", "返回执行结果"}."上传数据" ("枚举")) -> ()
          n286 = Equal To 0?(x=w466) -> (x = 0?=w467:bool)
          n287 = case shown="真" w467 {
            frame False {
            }
            frame True {
              n288 = global read "全局 小时数据发送次数.vi" "小时数据发送次数"() -> (w471:i32)
              n289 = Increment(x=w471) -> (x+1=w470:i32)
              n290 = global write "全局 小时数据发送次数.vi" "小时数据发送次数"(w470) -> ()
            }
          }
        }
        frame "上传数据" {
          n291 = global read "断电保存全局.vi" "数据发送协议"() -> (w473:enum16{"2005-212协议", "2017-212协议"})
          n292 = case shown="\"2017-212协议\", 默认" w473 {
            tunnel: ["" ("编码输出") w479] -> w472
            frame "2005-212协议" {
            }
            frame "2017-212协议", Default {
              (unwired) "w01010" ("污染物编码")
              (unwired) "w01016" ("污染物编码")
              (unwired) "w01003" ("污染物编码")
              (unwired) "w01009" ("污染物编码")
              (unwired) "w01001" ("污染物编码")
              (unwired) "w01014" ("污染物编码")
              (unwired) "w01100" ("污染物编码")
              # "时间,测量模式,数据类型,数据标识,层数,Temp,SpCond,Cond,Sal,TDS,pH,pHmV,ORP,ODO%,ODOmg/L,Turb,Chla,Depth,"
              n293 = global read "全局 小时数据发送次数.vi" "小时数据发送次数"() -> (w497:i32)
              n294 = global read "全局 所有参数.vi" "剖面多参数"() -> (w500:string[][])
              n295 = Index Array(array=w500, index (row)=w497) -> (element=w498:string[])  [unwired: 1 in]
              n296 = Index Array(array=w498, index #1=0 ("索引")) -> (element #1=w482:string, element #3=w496:string, element #4=w495:string, element #5=w494:string, element #6=w493:string, element #7=w492:string, element #11=w490:string, element #13=w489:string, element #15=w488:string, element #16=w487:string, element #17=w486:string)  [unwired: 16 in, 6 out]
              n297 = call "规范小时时间戳.vi"("字符串"=w482) -> ("result string"=w483:string)  [unwired: 10 in]
              n298 = Build Array(w493, w492, w490, w489, w488, w487, w486) -> (w491:string[])
              n299 = call "剖面多参数组合(子VI).vi"("数据类型实时小时"="-Avg=", "数据值"=w491, "层数"=w494, "数据标识"=w495, "数据类型"=w496) -> ("编码输出"=w478:string)  [unwired: 6 in]
              n300 = Format Into String(format string="DataTime=%s;", w483) -> (resulting string=w484:string)  [unwired: 2 in, 1 out]
              n301 = Empty String/Path?(string/path=w478) -> (empty?=w481:bool)
              n302 = Concatenate Strings(w484, w478) -> (w480:string)
              n303 = case shown="真" w481 {
                tunnel: [w501 ""] -> w479
                tunnel: w480 -> [w501 _]
                frame False {
                }
                frame True {
                }
              }
            }
          }
          n304 = Empty String/Path?(string/path=w472) -> (empty?=w475:bool)
          n305 = case shown="假" w475 {
            tunnel: [w505 ""] -> w474
            tunnel: w472 -> [w505 _]
            frame False {
              n306 = global read "全局 小时数据发送次数.vi" "小时数据发送次数"() -> (w504:i32)
              n307 = Increment(x=w504) -> (x+1=w503:i32)
              n308 = global write "全局 小时数据发送次数.vi" "小时数据发送次数"(w503) -> ()
            }
            frame True {
              n309 = global read "全局 小时数据发送次数.vi" "小时数据发送次数"() -> (w507:i32)
              n310 = Increment(x=w507) -> (x+1=w506:i32)
              n311 = global write "全局 小时数据发送次数.vi" "小时数据发送次数"(w506) -> ()
            }
          }
        }
        frame "返回执行结果" {
          (unwired) 0 ("当前包数")
          n312 = global write "全局1.vi" "枚举"(enum16{"返回请求应答", "上传数据", "返回执行结果"}."返回请求应答" ("枚举")) -> ()
        }
      }
    }
    frame "剖面多参数S" {
      # "发送实时数据"
      n313 = global read "全局1.vi" "枚举"() -> (w511:enum16{"返回请求应答", "上传数据", "返回执行结果"})
      n314 = case shown="\"上传数据\"" w511 {
        tunnel: ["QnRtn=1" w521 "ExeRtn=1"] -> w512
        frame "返回请求应答", Default {
          (unwired) 0 ("当前包数")
          n315 = global read "全局 数据数组大小.vi" "数据数组大小"() -> (w513:i32)
          n316 = global write "全局1.vi" "枚举"(enum16{"返回请求应答", "上传数据", "返回执行结果"}."上传数据" ("枚举")) -> ()
          n317 = Equal To 0?(x=w513) -> (x = 0?=w514:bool)
          n318 = case shown="真" w514 {
            frame False {
            }
            frame True {
              n319 = global read "全局 小时数据发送次数.vi" "小时数据发送次数"() -> (w518:i32)
              n320 = Increment(x=w518) -> (x+1=w517:i32)
              n321 = global write "全局 小时数据发送次数.vi" "小时数据发送次数"(w517) -> ()
            }
          }
        }
        frame "上传数据" {
          n322 = global read "断电保存全局.vi" "数据发送协议"() -> (w520:enum16{"2005-212协议", "2017-212协议"})
          n323 = case shown="\"2017-212协议\", 默认" w520 {
            tunnel: ["" ("编码输出") w528] -> w519
            frame "2005-212协议" {
            }
            frame "2017-212协议", Default {
              (unwired) "w01010" ("污染物编码")
              (unwired) "w01016" ("污染物编码")
              (unwired) "w01003" ("污染物编码")
              (unwired) "w01009" ("污染物编码")
              (unwired) "w01001" ("污染物编码")
              (unwired) "w01014" ("污染物编码")
              (unwired) "w01100" ("污染物编码")
              # "时间,测量模式,数据类型,数据标识,层数,Temp,SpCond,Cond,Sal,TDS,pH,pHmV,ORP,ODO%,ODOmg/L,Turb,Chla,Depth,"
              n324 = global read "全局 小时数据发送次数.vi" "小时数据发送次数"() -> (w544:i32)
              n325 = global read "全局 所有参数.vi" "剖面多参数"() -> (w547:string[][])
              n326 = Index Array(array=w547, index (row)=w544) -> (element=w545:string[])  [unwired: 1 in]
              n327 = Index Array(array=w545, index #1=0 ("索引")) -> (element #1=w525:string, element #3=w543:string, element #4=w542:string, element #5=w541:string, element #6=w540:string, element #7=w539:string, element #11=w537:string, element #13=w536:string, element #15=w535:string, element #16=w534:string, element #17=w533:string)  [unwired: 16 in, 6 out]
              n328 = call "规范时间戳.vi"("字符串"=w525) -> ("result string"=w524:string)  [unwired: 10 in]
              n329 = Build Array(w540, w539, w537, w536, w535, w534, w533) -> (w538:string[])
              n330 = call "剖面多参数组合(子VI).vi"("数据类型实时小时"="-Rtd=", "数据值"=w538, "层数"=w541, "数据标识"=w542, "数据类型"=w543) -> ("编码输出"=w527:string)  [unwired: 6 in]
              n331 = Format Into String(format string="DataTime=%s;", w524) -> (resulting string=w531:string)  [unwired: 2 in, 1 out]
              n332 = Empty String/Path?(string/path=w527) -> (empty?=w530:bool)
              n333 = Concatenate Strings(w531, w527) -> (w529:string)
              n334 = case shown="假" w530 {
                tunnel: [w548 ""] -> w528
                tunnel: w529 -> [w548 _]
                frame False {
                }
                frame True {
                }
              }
            }
          }
          n335 = Empty String/Path?(string/path=w519) -> (empty?=w522:bool)
          n336 = case shown="假" w522 {
            tunnel: [w552 ""] -> w521
            tunnel: w519 -> [w552 _]
            frame False {
              n337 = global read "全局 小时数据发送次数.vi" "小时数据发送次数"() -> (w551:i32)
              n338 = Increment(x=w551) -> (x+1=w550:i32)
              n339 = global write "全局 小时数据发送次数.vi" "小时数据发送次数"(w550) -> ()
            }
            frame True {
              n340 = global read "全局 小时数据发送次数.vi" "小时数据发送次数"() -> (w554:i32)
              n341 = Increment(x=w554) -> (x+1=w553:i32)
              n342 = global write "全局 小时数据发送次数.vi" "小时数据发送次数"(w553) -> ()
            }
          }
        }
        frame "返回执行结果" {
          (unwired) 0 ("当前包数")
          n343 = global write "全局1.vi" "枚举"(enum16{"返回请求应答", "上传数据", "返回执行结果"}."返回请求应答" ("枚举")) -> ()
        }
      }
    }
    frame "提取小时数据" {
      # "发送小时数据"
      n344 = global read "全局 小时数据发送次数.vi" "小时数据发送次数"() -> (w560:i32)
      n345 = Index Array(array=w562, index (row)=w560) -> (element=w559:string[])  [unwired: 1 in]
      n346 = global read "全局1.vi" "枚举"() -> (w561:enum16{"返回请求应答", "上传数据", "返回执行结果"})
      n347 = case shown="\"上传数据\"" w561 {
        tunnel: ["QnRtn=1" w577 "ExeRtn=1"] -> w563
        tunnel: w559 -> [_ w579 _]
        tunnel: w558 -> [_ w569 _]
        frame "返回请求应答", Default {
          n348 = global read "全局 数据数组大小.vi" "数据数组大小"() -> (w564:i32)
          n349 = Equal To 0?(x=w564) -> (x = 0?=w565:bool)
          n350 = case shown="真" w565 {
            frame False {
            }
            frame True {
              n351 = global read "全局 小时数据发送次数.vi" "小时数据发送次数"() -> (w568:i32)
              n352 = Increment(x=w568) -> (x+1=w567:i32)
              n353 = global write "全局 小时数据发送次数.vi" "小时数据发送次数"(w567) -> ()
            }
          }
        }
        frame "上传数据" {
          n354 = Index Array(array=w579, index #2=1 ("索引")) -> (element #1=w572:string)  [unwired: 1 in, 1 out]
          n355 = call "规范小时时间戳.vi"("字符串"=w572) -> ("result string"=w573:string)  [unwired: 10 in]
          n356 = call "数据发送组合-20200825 (子VI).vi"("枚举"=T4."提取小时数据", "插值后的数组元素"=w569) -> ("字符串"=w570:string)  [unwired: 9 in]
          n357 = Format Into String(format string="DataTime=%s;", w573) -> (resulting string=w576:string)  [unwired: 2 in, 1 out]
          n358 = Empty String/Path?(string/path=w570) -> (empty?=w578:bool)
          n359 = Concatenate Strings(w576, w570) -> (w574:string)
          n360 = case shown="假" w578 {
            tunnel: [w583 ""] -> w577
            tunnel: w574 -> [w583 _]
            frame False {
              n361 = global read "全局 小时数据发送次数.vi" "小时数据发送次数"() -> (w582:i32)
              n362 = Increment(x=w582) -> (x+1=w581:i32)
              n363 = global write "全局 小时数据发送次数.vi" "小时数据发送次数"(w581) -> ()
            }
            frame True {
              n364 = global read "全局 小时数据发送次数.vi" "小时数据发送次数"() -> (w585:i32)
              n365 = Increment(x=w585) -> (x+1=w584:i32)
              n366 = global write "全局 小时数据发送次数.vi" "小时数据发送次数"(w584) -> ()
            }
          }
        }
        frame "返回执行结果" {
        }
      }
    }
    frame "提取实时数据" {
      # "提取实时数据"
      n367 = global read "全局 小时数据发送次数.vi" "小时数据发送次数"() -> (w590:i32)
      n368 = Index Array(array=w593, index (row)=w590) -> (element=w589:string[])  [unwired: 1 in]
      n369 = global read "全局1.vi" "枚举"() -> (w591:enum16{"返回请求应答", "上传数据", "返回执行结果"})
      n370 = case shown="\"上传数据\"" w591 {
        tunnel: ["QnRtn=1" w602 "ExeRtn=1"] -> w592
        tunnel: w589 -> [_ w608 _]
        tunnel: w588 -> [_ w600 _]
        frame "返回请求应答", Default {
          n371 = global read "全局 数据数组大小.vi" "数据数组大小"() -> (w594:i32)
          n372 = Equal To 0?(x=w594) -> (x = 0?=w595:bool)
          n373 = case shown="真" w595 {
            frame False {
            }
            frame True {
              n374 = global read "全局 小时数据发送次数.vi" "小时数据发送次数"() -> (w598:i32)
              n375 = Increment(x=w598) -> (x+1=w597:i32)
              n376 = global write "全局 小时数据发送次数.vi" "小时数据发送次数"(w597) -> ()
            }
          }
        }
        frame "上传数据" {
          n377 = Index Array(array=w608, index #1=0 ("索引"), index #2=3 ("索引"), index #3=5 ("索引")) -> (element #1=w606:string)  [unwired: 2 out]
          n378 = call "规范时间戳.vi"("字符串"=w606) -> ("result string"=w605:string)  [unwired: 10 in]
          n379 = call "数据发送组合-20200825 (子VI).vi"("枚举"=T4."提取实时数据", "插值后的数组元素"=w600) -> ("字符串"=w599:string)  [unwired: 9 in]
          n380 = Empty String/Path?(string/path=w605) -> (empty?=w604:bool)
          n381 = Format Into String(format string="DataTime=%s;%s" ("格式字符串"), w605, w599) -> (resulting string=w603:string)  [unwired: 2 in, 1 out]
          n382 = case shown="真" w604 {
            tunnel: [w612 ""] -> w602
            tunnel: w603 -> [w612 _]
            frame False {
              n383 = global read "全局 小时数据发送次数.vi" "小时数据发送次数"() -> (w614:i32)
              n384 = Increment(x=w614) -> (x+1=w613:i32)
              n385 = global write "全局 小时数据发送次数.vi" "小时数据发送次数"(w613) -> ()
            }
            frame True {
              n386 = global read "全局 小时数据发送次数.vi" "小时数据发送次数"() -> (w616:i32)
              n387 = Increment(x=w616) -> (x+1=w615:i32)
              n388 = global write "全局 小时数据发送次数.vi" "小时数据发送次数"(w615) -> ()
            }
          }
        }
        frame "返回执行结果" {
        }
      }
    }
    frame "核查数据" {
      # "提取标样核查数据"
      n389 = global read "全局 小时数据发送次数.vi" "小时数据发送次数"() -> (w622:i32)
      n390 = Index Array(array=w619, index (row)=w622) -> (element=w621:string[])  [unwired: 1 in]
      n391 = global read "全局1.vi" "枚举"() -> (w623:enum16{"返回请求应答", "上传数据", "返回执行结果"})
      n392 = case shown="\"上传数据\"" w623 {
        tunnel: ["QnRtn=1" w635 "ExeRtn=1"] -> w624
        tunnel: w621 -> [_ w641 _]
        tunnel: w620 -> [_ w631 _]
        frame "返回请求应答", Default {
          n393 = global read "全局 数据数组大小.vi" "数据数组大小"() -> (w626:i32)
          n394 = Equal To 0?(x=w626) -> (x = 0?=w625:bool)
          n395 = case shown="真" w625 {
            frame False {
            }
            frame True {
              n396 = global read "全局 小时数据发送次数.vi" "小时数据发送次数"() -> (w629:i32)
              n397 = Increment(x=w629) -> (x+1=w628:i32)
              n398 = global write "全局 小时数据发送次数.vi" "小时数据发送次数"(w628) -> ()
            }
          }
        }
        frame "上传数据" {
          # "将非空数组的时间戳写入"
          n399 = Index Array(array=w641, index #1=0 ("索引"), index #2=3 ("索引"), index #3=7 ("索引")) -> (element #1=w634:string)  [unwired: 2 out]
          n400 = call "数据发送组合-20200825 (子VI).vi"("枚举"=T4."核查数据", "插值后的数组元素"=w631) -> ("字符串"=w630:string)  [unwired: 9 in]
          n401 = call "规范时间戳.vi"("字符串"=w634) -> ("result string"=w633:string)  [unwired: 10 in]
          n402 = Empty String/Path?(string/path=w633) -> (empty?=w637:bool)
          n403 = Format Into String(format string="DataTime=%s;%s" ("格式字符串"), w633, w630) -> (resulting string=w636:string)  [unwired: 2 in, 1 out]
          n404 = case shown="假" w637 {
            tunnel: [w645 ""] -> w635
            tunnel: w636 -> [w645 _]
            frame False {
              n405 = global read "全局 小时数据发送次数.vi" "小时数据发送次数"() -> (w644:i32)
              n406 = Increment(x=w644) -> (x+1=w643:i32)
              n407 = global write "全局 小时数据发送次数.vi" "小时数据发送次数"(w643) -> ()
            }
            frame True {
              n408 = global read "全局 小时数据发送次数.vi" "小时数据发送次数"() -> (w647:i32)
              n409 = Increment(x=w647) -> (x+1=w646:i32)
              n410 = global write "全局 小时数据发送次数.vi" "小时数据发送次数"(w646) -> ()
            }
          }
        }
        frame "返回执行结果" {
        }
      }
    }
    frame "空白测试", "跨度核查", "零点核查" {
      # "提取空白测试数据/零点核查数据/跨度核查数据"
      n411 = global read "全局 小时数据发送次数.vi" "小时数据发送次数"() -> (w653:i32)
      n412 = Index Array(array=w650, index (row)=w653) -> (element=w652:string[])  [unwired: 1 in]
      n413 = global read "全局1.vi" "枚举"() -> (w654:enum16{"返回请求应答", "上传数据", "返回执行结果"})
      n414 = case shown="\"上传数据\"" w654 {
        tunnel: ["QnRtn=1" w666 "ExeRtn=1"] -> w655
        tunnel: w652 -> [_ w671 _]
        tunnel: w651 -> [_ w662 _]
        frame "返回请求应答", Default {
          (unwired) 0 ("当前包数")
          n415 = global read "全局 数据数组大小.vi" "数据数组大小"() -> (w657:i32)
          n416 = Equal To 0?(x=w657) -> (x = 0?=w656:bool)
          n417 = case shown="真" w656 {
            frame False {
            }
            frame True {
              n418 = global read "全局 小时数据发送次数.vi" "小时数据发送次数"() -> (w660:i32)
              n419 = Increment(x=w660) -> (x+1=w659:i32)
              n420 = global write "全局 小时数据发送次数.vi" "小时数据发送次数"(w659) -> ()
            }
          }
        }
        frame "上传数据" {
          # "将非空数组的时间戳写入"
          n421 = Index Array(array=w671, index #1=0 ("索引"), index #2=3 ("索引")) -> (element #1=w665:string)  [unwired: 1 out]
          n422 = call "数据发送组合-20200825 (子VI).vi"("枚举"=T4."空白零点跨度数据", "插值后的数组元素"=w662) -> ("字符串"=w661:string)  [unwired: 9 in]
          n423 = call "规范时间戳.vi"("字符串"=w665) -> ("result string"=w664:string)  [unwired: 10 in]
          n424 = Empty String/Path?(string/path=w664) -> (empty?=w668:bool)
          n425 = Format Into String(format string="DataTime=%s;%s" ("格式字符串"), w664, w661) -> (resulting string=w667:string)  [unwired: 2 in, 1 out]
          n426 = case shown="假" w668 {
            tunnel: [w675 ""] -> w666
            tunnel: w667 -> [w675 _]
            frame False {
              n427 = global read "全局 小时数据发送次数.vi" "小时数据发送次数"() -> (w674:i32)
              n428 = Increment(x=w674) -> (x+1=w673:i32)
              n429 = global write "全局 小时数据发送次数.vi" "小时数据发送次数"(w673) -> ()
            }
            frame True {
              n430 = global read "全局 小时数据发送次数.vi" "小时数据发送次数"() -> (w677:i32)
              n431 = Increment(x=w677) -> (x+1=w676:i32)
              n432 = global write "全局 小时数据发送次数.vi" "小时数据发送次数"(w676) -> ()
            }
          }
        }
        frame "返回执行结果" {
        }
      }
    }
    frame "提取加标回收" {
      # "提取加标回收数据"
      n433 = global read "全局1.vi" "枚举"() -> (w683:enum16{"返回请求应答", "上传数据", "返回执行结果"})
      n434 = case shown="\"上传数据\"" w683 {
        tunnel: ["QnRtn=1" w695 "ExeRtn=1"] -> w681
        tunnel: w682 -> [_ w697 _]
        tunnel: w680 -> [_ w689 _]
        frame "返回请求应答", Default {
          n435 = global read "全局 数据数组大小.vi" "数据数组大小"() -> (w684:i32)
          n436 = Equal To 0?(x=w684) -> (x = 0?=w685:bool)
          n437 = case shown="真" w685 {
            frame False {
            }
            frame True {
              n438 = global read "全局 小时数据发送次数.vi" "小时数据发送次数"() -> (w688:i32)
              n439 = Increment(x=w688) -> (x+1=w687:i32)
              n440 = global write "全局 小时数据发送次数.vi" "小时数据发送次数"(w687) -> ()
            }
          }
        }
        frame "上传数据" {
          # "w01001-Check=63.0,w01001-WaterTime=20160801080000,w01001-Water=45.23,w01001-Chroma=1000,w01001-Volume=0.2,w01001-DVolume=200,w01003-Flag=N;"
          # "CODMn"
          n441 = global read "全局 小时数据发送次数.vi" "小时数据发送次数"() -> (w692:i32)
          n442 = call "数据发送组合-20200825 (子VI).vi"("枚举"=T4."加标回收测试", "插值后的数组元素"=w689) -> ("字符串"=w690:string)  [unwired: 9 in]
          n443 = call "加标回收数据组合 (子VI).vi"("小时数据发送次数"=w692, "数据"=w697, "污染物编码"="w01019") -> ("datatime"=w699:string)  [unwired: 7 in, 1 out]
          n444 = call "规范时间戳.vi"("字符串"=w699) -> ("result string"=w698:string)  [unwired: 10 in]
          n445 = Empty String/Path?(string/path=w698) -> (empty?=w694:bool)
          n446 = Format Into String(format string="DataTime=%s;%s" ("格式字符串"), w698, w690) -> (resulting string=w696:string)  [unwired: 2 in, 1 out]
          n447 = case shown="真" w694 {
            tunnel: [w703 ""] -> w695
            tunnel: w696 -> [w703 _]
            frame False {
              n448 = global read "全局 小时数据发送次数.vi" "小时数据发送次数"() -> (w702:i32)
              n449 = Increment(x=w702) -> (x+1=w701:i32)
              n450 = global write "全局 小时数据发送次数.vi" "小时数据发送次数"(w701) -> ()
            }
            frame True {
              n451 = global read "全局 小时数据发送次数.vi" "小时数据发送次数"() -> (w705:i32)
              n452 = Increment(x=w705) -> (x+1=w704:i32)
              n453 = global write "全局 小时数据发送次数.vi" "小时数据发送次数"(w704) -> ()
            }
          }
        }
        frame "返回执行结果" {
        }
      }
    }
    frame "提取平行样" {
      # "提取平行样数据"
      n454 = global read "全局1.vi" "枚举"() -> (w711:enum16{"返回请求应答", "上传数据", "返回执行结果"})
      n455 = case shown="\"上传数据\"" w711 {
        tunnel: ["QnRtn=1" w727 "ExeRtn=1"] -> w710
        tunnel: w709 -> [_ w721 _]
        tunnel: w708 -> [_ w717 _]
        frame "返回请求应答", Default {
          n456 = global read "全局 数据数组大小.vi" "数据数组大小"() -> (w712:i32)
          n457 = Equal To 0?(x=w712) -> (x = 0?=w713:bool)
          n458 = case shown="真" w713 {
            frame False {
            }
            frame True {
              n459 = global read "全局 小时数据发送次数.vi" "小时数据发送次数"() -> (w716:i32)
              n460 = Increment(x=w716) -> (x+1=w715:i32)
              n461 = global write "全局 小时数据发送次数.vi" "小时数据发送次数"(w715) -> ()
            }
          }
        }
        frame "上传数据" {
          # "CODMn"
          n462 = global read "全局 小时数据发送次数.vi" "小时数据发送次数"() -> (w720:i32)
          n463 = call "数据发送组合-20200825 (子VI).vi"("枚举"=T4."平行样测试", "插值后的数组元素"=w717) -> ("字符串"=w718:string)  [unwired: 9 in]
          n464 = Index Array(array=w721, index (row)=w720) -> (element=w725:string[])  [unwired: 1 in]
          n465 = Index Array(array=w725, index=0 ("索引")) -> (element=w722:string)
          n466 = call "规范时间戳.vi"("字符串"=w722) -> ("result string"=w723:string)  [unwired: 10 in]
          n467 = Empty String/Path?(string/path=w722) -> (empty?=w726:bool)
          n468 = Format Into String(format string="DataTime=%s;%s" ("格式字符串"), w723, w718) -> (resulting string=w728:string)  [unwired: 2 in, 1 out]
          n469 = case shown="真" w726 {
            tunnel: [w732 ""] -> w727
            tunnel: w728 -> [w732 _]
            frame False {
              n470 = global read "全局 小时数据发送次数.vi" "小时数据发送次数"() -> (w731:i32)
              n471 = Increment(x=w731) -> (x+1=w730:i32)
              n472 = global write "全局 小时数据发送次数.vi" "小时数据发送次数"(w730) -> ()
            }
            frame True {
              n473 = global read "全局 小时数据发送次数.vi" "小时数据发送次数"() -> (w734:i32)
              n474 = Increment(x=w734) -> (x+1=w733:i32)
              n475 = global write "全局 小时数据发送次数.vi" "小时数据发送次数"(w733) -> ()
            }
          }
        }
        frame "返回执行结果" {
        }
      }
    }
    frame "提取集成干预" {
      # "提取平行样数据"
      n476 = global read "全局1.vi" "枚举"() -> (w740:enum16{"返回请求应答", "上传数据", "返回执行结果"})
      n477 = case shown="\"上传数据\"" w740 {
        tunnel: ["QnRtn=1" w757 "ExeRtn=1"] -> w739
        tunnel: w738 -> [_ w752 _]
        tunnel: w737 -> [_ w749 _]
        frame "返回请求应答", Default {
          n478 = global read "全局 数据数组大小.vi" "数据数组大小"() -> (w741:i32)
          n479 = Equal To 0?(x=w741) -> (x = 0?=w742:bool)
          n480 = case shown="真" w742 {
            frame False {
            }
            frame True {
              n481 = global read "全局 小时数据发送次数.vi" "小时数据发送次数"() -> (w745:i32)
              n482 = Increment(x=w745) -> (x+1=w744:i32)
              n483 = global write "全局 小时数据发送次数.vi" "小时数据发送次数"(w744) -> ()
            }
          }
        }
        frame "上传数据" {
          # "CODMn"
          n484 = global read "全局 小时数据发送次数.vi" "小时数据发送次数"() -> (w753:i32)
          n485 = call "数据发送组合-20200825 (子VI).vi"("枚举"=T4."集成干预测试", "插值后的数组元素"=w749) -> ("字符串"=w750:string)  [unwired: 9 in]
          n486 = Index Array(array=w752, index (row)=w753) -> (element=w755:string[])  [unwired: 1 in]
          n487 = global read "断电保存全局.vi" "应用环境"() -> (w748:enum16{"STD", "GB212"})
          n488 = Index Array(array=w755, index=0 ("索引")) -> (element=w747:string)
          n489 = case shown="\"STD\", 默认" w748 {
            tunnel: [w761 w762] -> w746
            tunnel: w747 -> [w760 w763]
            frame "STD", Default {
              n490 = call "规范时间戳.vi"("字符串"=w760) -> ("result string"=w761:string)  [unwired: 10 in]
            }
            frame "GB212" {
              n491 = call "规范分钟数据时间戳.vi"("字符串"=w763) -> ("result string"=w762:string)  [unwired: 10 in]
            }
          }
          n492 = Empty String/Path?(string/path=w747) -> (empty?=w756:bool)
          n493 = Format Into String(format string="DataTime=%s;%s" ("格式字符串"), w746, w750) -> (resulting string=w758:string)  [unwired: 2 in, 1 out]
          n494 = case shown="真" w756 {
            tunnel: [w766 ""] -> w757
            tunnel: w758 -> [w766 _]
            frame False {
              n495 = global read "全局 小时数据发送次数.vi" "小时数据发送次数"() -> (w765:i32)
              n496 = Increment(x=w765) -> (x+1=w764:i32)
              n497 = global write "全局 小时数据发送次数.vi" "小时数据发送次数"(w764) -> ()
            }
            frame True {
              n498 = global read "全局 小时数据发送次数.vi" "小时数据发送次数"() -> (w768:i32)
              n499 = Increment(x=w768) -> (x+1=w767:i32)
              n500 = global write "全局 小时数据发送次数.vi" "小时数据发送次数"(w767) -> ()
            }
          }
        }
        frame "返回执行结果" {
        }
      }
    }
    frame "操作日志" {
      n501 = global read "全局 小时数据发送次数.vi" "小时数据发送次数"() -> (w773:i32)
      n502 = Index Array(array=w775, index (row)=w773) -> (element=w772:string[])  [unwired: 1 in]
      n503 = global read "全局1.vi" "枚举"() -> (w774:enum16{"返回请求应答", "上传数据", "返回执行结果"})
      n504 = case shown="\"上传数据\"" w774 {
        tunnel: ["QnRtn=1" w793 "ExeRtn=1"] -> w776
        tunnel: w772 -> [_ w795 _]
        tunnel: w771 -> [_ w783 _]
        frame "返回请求应答", Default {
          n505 = global read "全局 数据数组大小.vi" "数据数组大小"() -> (w779:i32)
          n506 = Equal To 0?(x=w779) -> (x = 0?=w778:bool)
          n507 = case shown="真" w778 {
            frame False {
            }
            frame True {
              n508 = global read "全局 小时数据发送次数.vi" "小时数据发送次数"() -> (w781:i32)
              n509 = Increment(x=w781) -> (x+1=w780:i32)
              n510 = global write "全局 小时数据发送次数.vi" "小时数据发送次数"(w780) -> ()
            }
          }
        }
        frame "上传数据" {
          n511 = Index Array(array=w795, index #1=0 ("索引"), index #2=2 ("索引")) -> (element #1=w788:string)  [unwired: 1 out]
          n512 = call "规范时间戳.vi"("字符串"=w788) -> ("result string"=w786:string)  [unwired: 10 in]
          n513 = call "数据发送组合-20200825 (子VI).vi"("枚举"=T5."操作日志", "插值后的数组元素"=w783) -> ("字符串"=w782:string)  [unwired: 9 in]
          n514 = Format Into String(format string="DataTime=%s;", w786) -> (resulting string=w785:string)  [unwired: 2 in, 1 out]
          n515 = Concatenate Strings(w785, w782) -> (w790:string)
          n516 = Empty String/Path?(string/path=w790) -> (empty?=w794:bool)
          n517 = String Length(string=w790) -> (length=w792:i32)
          n518 = Decrement(x=w792) -> (x-1=w791:i32)
          n519 = String Subset(string=w790, length (rest)=w791) -> (substring=w789:string)  [unwired: 1 in]
          n520 = case shown="假" w794 {
            tunnel: [w800 ""] -> w793
            tunnel: w789 -> [w800 _]
            frame False {
              n521 = global read "全局 小时数据发送次数.vi" "小时数据发送次数"() -> (w799:i32)
              n522 = Increment(x=w799) -> (x+1=w798:i32)
              n523 = global write "全局 小时数据发送次数.vi" "小时数据发送次数"(w798) -> ()
            }
            frame True {
              n524 = global read "全局 小时数据发送次数.vi" "小时数据发送次数"() -> (w802:i32)
              n525 = Increment(x=w802) -> (x+1=w801:i32)
              n526 = global write "全局 小时数据发送次数.vi" "小时数据发送次数"(w801) -> ()
            }
          }
        }
        frame "返回执行结果" {
        }
      }
    }
    frame "仪器参数" {
      n527 = global read "全局 小时数据发送次数.vi" "小时数据发送次数"() -> (w807:i32)
      n528 = Index Array(array=w809, index (row)=w807) -> (element=w806:string[])  [unwired: 1 in]
      n529 = global read "全局1.vi" "枚举"() -> (w808:enum16{"返回请求应答", "上传数据", "返回执行结果"})
      n530 = case shown="\"上传数据\"" w808 {
        tunnel: ["QnRtn=1" w827 "ExeRtn=1"] -> w810
        tunnel: w806 -> [_ w825 _]
        tunnel: w805 -> [_ w819 _]
        frame "返回请求应答", Default {
          n531 = global read "全局 数据数组大小.vi" "数据数组大小"() -> (w813:i32)
          n532 = Equal To 0?(x=w813) -> (x = 0?=w812:bool)
          n533 = case shown="真" w812 {
            frame False {
            }
            frame True {
              n534 = global read "全局 小时数据发送次数.vi" "小时数据发送次数"() -> (w815:i32)
              n535 = Increment(x=w815) -> (x+1=w814:i32)
              n536 = global write "全局 小时数据发送次数.vi" "小时数据发送次数"(w814) -> ()
            }
          }
        }
        frame "上传数据" {
          n537 = Index Array(array=w825) -> (element=w816:string)  [unwired: 1 in]
          n538 = call "规范小时时间戳.vi"("字符串"=w816) -> ("result string"=w817:string)  [unwired: 10 in]
          n539 = call "数据发送组合-20200825 (子VI).vi"("枚举"=T6."仪器参数", "插值后的数组元素"=w819) -> ("字符串"=w818:string)  [unwired: 9 in]
          n540 = Format Into String(format string="DataTime=%s;%s" ("格式字符串"), w817, w818) -> (resulting string=w822:string)  [unwired: 2 in, 1 out]
          n541 = String Length(string=w822) -> (length=w823:i32)
          n542 = Decrement(x=w823) -> (x-1=w824:i32)
          n543 = String Subset(string=w822, length (rest)=w824) -> (substring=w821:string)  [unwired: 1 in]
          n544 = Empty String/Path?(string/path=w821) -> (empty?=w828:bool)
          n545 = case shown="假" w828 {
            tunnel: [w831 ""] -> w827
            tunnel: w821 -> [w831 _]
            frame False {
              n546 = global read "全局 小时数据发送次数.vi" "小时数据发送次数"() -> (w830:i32)
              n547 = Increment(x=w830) -> (x+1=w829:i32)
              n548 = global write "全局 小时数据发送次数.vi" "小时数据发送次数"(w829) -> ()
            }
            frame True {
              n549 = global read "全局 小时数据发送次数.vi" "小时数据发送次数"() -> (w833:i32)
              n550 = Increment(x=w833) -> (x+1=w832:i32)
              n551 = global write "全局 小时数据发送次数.vi" "小时数据发送次数"(w832) -> ()
            }
          }
        }
        frame "返回执行结果" {
        }
      }
    }
    frame "3090仪器参数" {
      n552 = global read "全局 小时数据发送次数.vi" "小时数据发送次数"() -> (w838:i32)
      n553 = Index Array(array=w840, index (row)=w838) -> (element=w837:string[])  [unwired: 1 in]
      n554 = global read "全局1.vi" "枚举"() -> (w839:enum16{"返回请求应答", "上传数据", "返回执行结果"})
      n555 = case shown="\"上传数据\"" w839 {
        tunnel: ["QnRtn=1" w858 "ExeRtn=1"] -> w841
        tunnel: w837 -> [_ w855 _]
        tunnel: w836 -> [_ w848 _]
        frame "返回请求应答", Default {
          n556 = global read "全局 数据数组大小.vi" "数据数组大小"() -> (w844:i32)
          n557 = Equal To 0?(x=w844) -> (x = 0?=w843:bool)
          n558 = case shown="真" w843 {
            frame False {
            }
            frame True {
              n559 = global read "全局 小时数据发送次数.vi" "小时数据发送次数"() -> (w846:i32)
              n560 = Increment(x=w846) -> (x+1=w845:i32)
              n561 = global write "全局 小时数据发送次数.vi" "小时数据发送次数"(w845) -> ()
            }
          }
        }
        frame "上传数据" {
          n562 = Index Array(array=w855) -> (element=w854:string)  [unwired: 1 in]
          n563 = call "规范时间戳.vi"("字符串"=w854) -> ("result string"=w856:string)  [unwired: 10 in]
          n564 = call "数据发送组合-20200825 (子VI).vi"("枚举"=T6."3090仪器参数", "插值后的数组元素"=w848) -> ("字符串"=w847:string)  [unwired: 9 in]
          n565 = Format Into String(format string="DataTime=%s;%s" ("格式字符串"), w856, w847) -> (resulting string=w851:string)  [unwired: 2 in, 1 out]
          n566 = String Length(string=w851) -> (length=w852:i32)
          n567 = Decrement(x=w852) -> (x-1=w853:i32)
          n568 = String Subset(string=w851, length (rest)=w853) -> (substring=w850:string)  [unwired: 1 in]
          n569 = Empty String/Path?(string/path=w850) -> (empty?=w859:bool)
          n570 = case shown="假" w859 {
            tunnel: [w862 ""] -> w858
            tunnel: w850 -> [w862 _]
            frame False {
              n571 = global read "全局 小时数据发送次数.vi" "小时数据发送次数"() -> (w861:i32)
              n572 = Increment(x=w861) -> (x+1=w860:i32)
              n573 = global write "全局 小时数据发送次数.vi" "小时数据发送次数"(w860) -> ()
            }
            frame True {
              n574 = global read "全局 小时数据发送次数.vi" "小时数据发送次数"() -> (w864:i32)
              n575 = Increment(x=w864) -> (x+1=w863:i32)
              n576 = global write "全局 小时数据发送次数.vi" "小时数据发送次数"(w863) -> ()
            }
          }
        }
        frame "返回执行结果" {
        }
      }
    }
    frame "提取仪器参数" {
      n577 = global read "全局1.vi" "枚举"() -> (w868:enum16{"返回请求应答", "上传数据", "返回执行结果"})
      n578 = case shown="\"上传数据\"" w868 {
        tunnel: ["QnRtn=1" w878 "ExeRtn=1"] -> w869
        tunnel: w867 -> [_ w876 _]
        frame "返回请求应答", Default {
          n579 = global read "全局 数据数组大小.vi" "数据数组大小"() -> (w872:i32)
          n580 = Equal To 0?(x=w872) -> (x = 0?=w871:bool)
          n581 = case shown="假" w871 {
            frame False {
            }
            frame True {
              n582 = global read "全局 小时数据发送次数.vi" "小时数据发送次数"() -> (w874:i32)
              n583 = Increment(x=w874) -> (x+1=w873:i32)
              n584 = global write "全局 小时数据发送次数.vi" "小时数据发送次数"(w873) -> ()
            }
          }
        }
        frame "上传数据" {
          n585 = call "数据发送组合-20200825 (子VI).vi"("枚举"=T6."提取仪器参数", "插值后的数组元素"=w876) -> ("字符串"=w875:string)  [unwired: 9 in]
          n586 = Empty String/Path?(string/path=w875) -> (empty?=w879:bool)
          n587 = case shown="假" w879 {
            tunnel: [w882 ""] -> w878
            tunnel: w875 -> [w882 _]
            frame False {
              n588 = global read "全局 小时数据发送次数.vi" "小时数据发送次数"() -> (w881:i32)
              n589 = Increment(x=w881) -> (x+1=w880:i32)
              n590 = global write "全局 小时数据发送次数.vi" "小时数据发送次数"(w880) -> ()
            }
            frame True {
              n591 = global read "全局 小时数据发送次数.vi" "小时数据发送次数"() -> (w884:i32)
              n592 = Increment(x=w884) -> (x+1=w883:i32)
              n593 = global write "全局 小时数据发送次数.vi" "小时数据发送次数"(w883) -> ()
            }
          }
        }
        frame "返回执行结果" {
        }
      }
    }
    frame "报警信息" {
      n594 = global read "全局 小时数据发送次数.vi" "小时数据发送次数"() -> (w889:i32)
      n595 = Index Array(array=w891, index (row)=w889) -> (element=w888:string[])  [unwired: 1 in]
      n596 = global read "全局1.vi" "枚举"() -> (w890:enum16{"返回请求应答", "上传数据", "返回执行结果"})
      n597 = case shown="\"上传数据\"" w890 {
        tunnel: ["QnRtn=1" w904 "ExeRtn=1"] -> w892
        tunnel: w888 -> [_ _ _]
        tunnel: w887 -> [_ w899 _]
        frame "返回请求应答", Default {
          n598 = global read "全局 数据数组大小.vi" "数据数组大小"() -> (w895:i32)
          n599 = Equal To 0?(x=w895) -> (x = 0?=w894:bool)
          n600 = case shown="真" w894 {
            frame False {
            }
            frame True {
              n601 = global read "全局 小时数据发送次数.vi" "小时数据发送次数"() -> (w897:i32)
              n602 = Increment(x=w897) -> (x+1=w896:i32)
              n603 = global write "全局 小时数据发送次数.vi" "小时数据发送次数"(w896) -> ()
            }
          }
        }
        frame "上传数据" {
          n604 = call "数据发送组合-20200825 (子VI).vi"("枚举"=T6."报警信息", "插值后的数组元素"=w899) -> ("字符串"=w898:string)  [unwired: 9 in]
          n605 = Empty String/Path?(string/path=w898) -> (empty?=w905:bool)
          n606 = String Length(string=w898) -> (length=w903:i32)
          n607 = Decrement(x=w903) -> (x-1=w902:i32)
          n608 = String Subset(string=w898, length (rest)=w902) -> (substring=w901:string)  [unwired: 1 in]
          n609 = case shown="假" w905 {
            tunnel: [w908 ""] -> w904
            tunnel: w901 -> [w908 _]
            frame False {
              n610 = global read "全局 小时数据发送次数.vi" "小时数据发送次数"() -> (w907:i32)
              n611 = Increment(x=w907) -> (x+1=w906:i32)
              n612 = global write "全局 小时数据发送次数.vi" "小时数据发送次数"(w906) -> ()
            }
            frame True {
              n613 = global read "全局 小时数据发送次数.vi" "小时数据发送次数"() -> (w910:i32)
              n614 = Increment(x=w910) -> (x+1=w909:i32)
              n615 = global write "全局 小时数据发送次数.vi" "小时数据发送次数"(w909) -> ()
            }
          }
        }
        frame "返回执行结果" {
        }
      }
    }
    frame "系统状态" {
      # ",i12002-Info=0,i12003-Info=100,i12031-Info=0"
      # "DataTime=20100301145000;PolId=w01018,i12001-Info=1,i12003-Info=100"
      # "100  当前模式\n101  CODMn状态  （0待机，1运行）\n102  氨氮状态\n103  总磷状态\n104  总氮状态\n105  CODCr状态\n106  运行周期"
      n616 = Get Date/Time In Seconds() -> (seconds since 1Jan1904=w930:timestamp)
      n617 = Format Date/Time String(time format string (%c)="%Y%m%d%H%M%S" ("时间格式字符串(%c)"), seconds (now)=w930) -> (date/time string=w929:string)  [unwired: 1 in]
      n618 = global read "全局 小时数据发送次数.vi" "小时数据发送次数"() -> (w917:i32)
      n619 = global read "全局1.vi" "register values"() -> (w918:u16[])
      n620 = Build Array("w00000", "w01019", "w21003", "w21011", "w21001", "w01018") -> (w920:string[])
      n621 = Index Array(array=w920, index=w917) -> (element=w919:string)
      n622 = Index Array(array=w918, index=w917) -> (element=w916:u16)
      n623 = case shown="1, 默认" w917 {
        tunnel: w919 -> [w935 w940]
        tunnel: w916 -> [w936 _]
        tunnel: [w933 w939] -> w915
        frame 1, Default {
          n624 = Number To Decimal String(number=w936) -> (decimal integer string=w937:string)  [unwired: 1 in]
          n625 = Format Into String(w937) -> (resulting string=w934:string)  [unwired: 3 in, 1 out]
          n626 = Format Into String(format string="PolId=%s,i12001-Info=%s,i12002-Info=0;" ("格式字符串"), w935, w934) -> (resulting string=w933:string)  [unwired: 2 in, 1 out]
        }
        frame 0 {
          n627 = Format Into String(format string="PolId=%s,i22001-Info=0,i22002-Info=1,i22003-Info=0;" ("格式字符串"), w940) -> (resulting string=w939:string)  [unwired: 2 in, 1 out]
        }
      }
      n628 = Format Into String(format string="DataTime=%s;%s" ("格式字符串"), w929, w915) -> (resulting string=w926:string)  [unwired: 2 in, 1 out]
      n629 = String Length(string=w926) -> (length=w928:i32)
      n630 = Decrement(x=w928) -> (x-1=w927:i32)
      n631 = String Subset(string=w926, length (rest)=w927) -> (substring=w925:string)  [unwired: 1 in]
    }
    frame "运行模式" {
      # "DataTime=20100301145000;PolId=w01018,i12001-Info=1,i12003-Info=0"
      # "100  当前模式\n101  CODMn状态  （0待机，1运行）\n102  氨氮状态\n103  总磷状态\n104  总氮状态\n105  CODCr状态\n106  运行周期"
      n632 = Get Date/Time In Seconds() -> (seconds since 1Jan1904=w949:timestamp)
      n633 = Format Date/Time String(time format string (%c)="%Y%m%d%H%M%S" ("时间格式字符串(%c)"), seconds (now)=w949) -> (date/time string=w946:string)  [unwired: 1 in]
      n634 = global read "全局1.vi" "register values"() -> (w951:u16[])
      n635 = Index Array(array=w951, index=0 ("索引")) -> (element=w943:u16)
      n636 = Number To Decimal String(number=w943) -> (decimal integer string=w945:string)  [unwired: 1 in]
      n637 = Format Into String(format string="RunMode=%s;" ("格式字符串"), w945) -> (resulting string=w942:string)  [unwired: 2 in, 1 out]
      n638 = Format Into String(format string="DataTime=%s;%s" ("格式字符串"), w946, w942) -> (resulting string=w948:string)  [unwired: 2 in, 1 out]
    }
    frame "测量周期" {
      # "DataTime=20100301145000;PolId=w01018,i12001-Info=1,i12003-Info=0"
      # "100  当前模式\n101  CODMn状态  （0待机，1运行）\n102  氨氮状态\n103  总磷状态\n104  总氮状态\n105  CODCr状态\n106  运行周期"
      n639 = global read "全局1.vi" "register values"() -> (w962:u16[])
      n640 = Get Date/Time In Seconds() -> (seconds since 1Jan1904=w960:timestamp)
      n641 = Format Date/Time String(time format string (%c)="%Y%m%d%H%M%S" ("时间格式字符串(%c)"), seconds (now)=w960) -> (date/time string=w957:string)  [unwired: 1 in]
      n642 = Index Array(array=w962, index=6 ("索引")) -> (element=w954:u16)
      n643 = Number To Decimal String(number=w954) -> (decimal integer string=w955:string)  [unwired: 1 in]
      n644 = Format Into String(format string="RunInterval=%s;" ("格式字符串"), w955) -> (resulting string=w953:string)  [unwired: 2 in, 1 out]
      n645 = Format Into String(format string="DataTime=%s;%s" ("格式字符串"), w957, w953) -> (resulting string=w959:string)  [unwired: 2 in, 1 out]
    }
    frame "超标留样" {
      # "DataTime=20100301145000;PolId=w01018,i12001-Info=1,i12003-Info=0"
      # "100  当前模式\n101  CODMn状态  （0待机，1运行）\n102  氨氮状态\n103  总磷状态\n104  总氮状态\n105  CODCr状态\n106  运行周期"
      n646 = global read "全局1.vi" "register values"() -> (w973:u16[])
      n647 = Get Date/Time In Seconds() -> (seconds since 1Jan1904=w971:timestamp)
      n648 = Format Date/Time String(time format string (%c)="%Y%m%d%H%M%S" ("时间格式字符串(%c)"), seconds (now)=w971) -> (date/time string=w968:string)  [unwired: 1 in]
      n649 = Index Array(array=w973, index=7 ("索引")) -> (element=w965:u16)
      n650 = Number To Decimal String(number=w965) -> (decimal integer string=w966:string)  [unwired: 1 in]
      n651 = Format Into String(format string="VaseNo=%s;" ("格式字符串"), w966) -> (resulting string=w964:string)  [unwired: 2 in, 1 out]
      n652 = Format Into String(format string="DataTime=%s;%s" ("格式字符串"), w968, w964) -> (resulting string=w970:string)  [unwired: 2 in, 1 out]
    }
  }
  n653 = case shown="假" w19 {
    tunnel: [w976 w980] -> w21
    frame False {
      n654 = global read "全局1.vi" "枚举"() -> (w975:enum16{"返回请求应答", "上传数据", "返回执行结果"})
      n655 = case shown="\"上传数据\"" w975 {
        tunnel: ["91" ("CN") w978 "91" ("CN")] -> w976
        frame "返回请求应答", Default {
        }
        frame "上传数据" {
          n656 = global read "全局1.vi" "系统编码ST"() -> (w978:string)
        }
        frame "返回执行结果" {
        }
      }
    }
    frame True {
      n657 = global read "全局 反控命令枚举.vi" "反控命令枚举"() -> (w981:enum16{"返回请求应答", "返回执行结果"})
      n658 = case shown="\"返回执行结果\"" w981 {
        tunnel: ["91" "91"] -> w980
        frame "返回请求应答", Default {
        }
        frame "返回执行结果" {
        }
      }
    }
  }
  n659 = case shown="\"心跳包\", 默认" "table输入" {
    tunnel: ["9015" ("ST") w994 w1002 w1010 w1017 w1024 w1032 w1040 w1049 w1064 w1072 w1080 w1089 w1098 w1115 w1123 w1131 w1139 w1147 w1155 w1166 w1178 w1186 "3020" ("ST") "3042" ("ST") "3056" ("ST") "3015" ("ST")] -> w24
    tunnel: ["9" ("ST") "8" ("ST") "8" ("ST") "8" ("ST") "8" ("ST") "8" ("ST") "8" ("ST") "8" ("ST") "9" ("ST") "9" ("ST") "9" ("ST") "9" ("ST") w1092 "8" ("ST") "9" ("ST") "8" ("ST") "8" ("ST") "9" ("ST") "9" ("ST") "8" ("ST") "9" ("ST") "9" ("ST") "8" ("ST") "9" ("ST") "9" ("ST") "9" ("ST") "9" ("ST")] -> w23
    tunnel: w13 -> [_ w992 w1000 w1011 w1018 w1025 w1033 w1041 w1050 w1066 w1074 w1082 w1091 w1101 w1117 w1125 w1133 w1141 w1149 w1157 w1168 w1180 w1188 w1194 w1198 w1202 w1206]
    tunnel: [_ w992 w1000 w1011 w1018 w1025 w1033 w1041 w1050 w1066 w1074 w1082 w1091 w1101 w1117 w1125 w1133 w1141 w1149 w1157 w1168 w1180 w1188 w1194 w1198 w1202 w1206] -> w2
    tunnel: [w984 w991 w999 w1007 w1015 w1022 w1030 w1038 w1046 w1063 w1071 w1079 w1088 w1100 w1113 w1121 w1129 w1137 w1145 w1153 w1161 w1173 w1185 w1193 w1197 w1201 w1205] -> w14
    frame "心跳包", Default {
      # "心跳包"
      n660 = Get Date/Time In Seconds() -> (seconds since 1Jan1904=w987:timestamp)
      n661 = Format Date/Time String(time format string (%c)="%Y%m%d%H%M%S%3u" ("时间格式字符串(%c)"), seconds (now)=w987) -> (date/time string=w986:string)  [unwired: 1 in]
      n662 = Search and Replace String(input string=w986, search string="." ("搜索字符串")) -> (result string=w984:string)  [unwired: 6 in, 3 out]
    }
    frame "提取数采仪时间" {
      n663 = global read "全局1.vi" "枚举"() -> (w995:enum16{"返回请求应答", "上传数据", "返回执行结果"})
      n664 = case shown="\"返回执行结果\"" w995 {
        tunnel: ["9011" ("CN") "1014" ("CN") "9012" ("CN")] -> w994
        frame "返回请求应答", Default {
        }
        frame "上传数据" {
        }
        frame "返回执行结果" {
        }
      }
      n665 = local read "QN"() -> (w991:string)
    }
    frame "提取实时数据间隔" {
      n666 = global read "全局1.vi" "枚举"() -> (w1003:enum16{"返回请求应答", "上传数据", "返回执行结果"})
      n667 = case shown="\"上传数据\"" w1003 {
        tunnel: ["9011" ("CN") "1061" ("CN") "9012" ("CN")] -> w1002
        frame "返回请求应答", Default {
        }
        frame "上传数据" {
        }
        frame "返回执行结果" {
        }
      }
      n668 = local read "QN"() -> (w999:string)
    }
    frame "反控命令" {
      n669 = global read "全局 反控命令枚举.vi" "反控命令枚举"() -> (w1008:enum16{"返回请求应答", "返回执行结果"})
      n670 = case shown="\"返回请求应答\", 默认" w1008 {
        tunnel: ["9011" ("CN") "9012" ("CN")] -> w1010
        frame "返回请求应答", Default {
        }
        frame "返回执行结果" {
        }
      }
      n671 = local read "QN"() -> (w1007:string)
    }
    frame "超标留样返回" {
      n672 = global read "全局1.vi" "枚举"() -> (w1014:enum16{"返回请求应答", "上传数据", "返回执行结果"})
      n673 = case shown="\"上传数据\"" w1014 {
        tunnel: ["9011" ("CN") "3015" ("CN") "9012" ("CN")] -> w1017
        frame "返回请求应答", Default {
        }
        frame "上传数据" {
        }
        frame "返回执行结果" {
        }
      }
      n674 = local read "QN"() -> (w1015:string)
    }
    frame "提取经纬度环境信息" {
      n675 = global read "全局1.vi" "枚举"() -> (w1026:enum16{"返回请求应答", "上传数据", "返回执行结果"})
      n676 = case shown="\"上传数据\"" w1026 {
        tunnel: ["9011" ("CN") "3041" ("CN") "9012" ("CN")] -> w1024
        frame "返回请求应答", Default {
        }
        frame "上传数据" {
        }
        frame "返回执行结果" {
        }
      }
      n677 = local read "QN"() -> (w1022:string)
    }
    frame "提取现场系统信息" {
      n678 = global read "全局1.vi" "枚举"() -> (w1034:enum16{"返回请求应答", "上传数据", "返回执行结果"})
      n679 = case shown="\"上传数据\"" w1034 {
        tunnel: ["9011" ("CN") "3040" ("CN") "9012" ("CN")] -> w1032
        frame "返回请求应答", Default {
        }
        frame "上传数据" {
        }
        frame "返回执行结果" {
        }
      }
      n680 = local read "QN"() -> (w1030:string)
    }
    frame "提取监测仪表时间" {
      n681 = global read "全局1.vi" "枚举"() -> (w1042:enum16{"返回请求应答", "上传数据", "返回执行结果"})
      n682 = case shown="\"返回执行结果\"" w1042 {
        tunnel: ["9011" ("CN") "1011" ("CN") "9012" ("CN")] -> w1040
        frame "返回请求应答", Default {
        }
        frame "上传数据" {
        }
        frame "返回执行结果" {
        }
      }
      n683 = local read "QN"() -> (w1038:string)
    }
    frame "实时数据" {
      n684 = global read "全局1.vi" "枚举"() -> (w1048:enum16{"返回请求应答", "上传数据", "返回执行结果"})
      n685 = case shown="\"上传数据\"" w1048 {
        tunnel: ["9011" ("CN") w1053 "9012" ("CN")] -> w1049
        frame "返回请求应答", Default {
        }
        frame "上传数据" {
          n686 = global read "全局 实时数据参数.vi" "实时数据参数"() -> (w1052:string)
          n687 = case shown="\"平行样测试\"" w1052 {
            tunnel: ["2011" ("CN") "2064" ("CN") "2082" ("CN") "2063" ("CN") "2062" ("CN") "2065" ("CN") "2066" ("CN") "fff" ("CN")] -> w1053
            frame "水样测试", Default {
            }
            frame "平行样测试" {
            }
            frame "集成干预测试" {
            }
            frame "加标回收测试" {
            }
            frame "核查数据" {
            }
            frame "空白测试" {
            }
            frame "跨度核查" {
            }
            frame "" {
            }
          }
        }
        frame "返回执行结果" {
        }
      }
      n688 = local read "QN"() -> (w1046:string)
    }
    frame "小时数据" {
      # "监测小时数据"
      n689 = global read "全局1.vi" "枚举"() -> (w1065:enum16{"返回请求应答", "上传数据", "返回执行结果"})
      n690 = case shown="\"上传数据\"" w1065 {
        tunnel: ["9011" ("CN") "2061" ("CN") "9012" ("CN")] -> w1064
        frame "返回请求应答", Default {
        }
        frame "上传数据" {
        }
        frame "返回执行结果" {
        }
      }
      n691 = local read "QN"() -> (w1063:string)
    }
    frame "剖面多参数H" {
      # "监测小时数据"
      n692 = global read "全局1.vi" "枚举"() -> (w1073:enum16{"返回请求应答", "上传数据", "返回执行结果"})
      n693 = case shown="\"上传数据\"" w1073 {
        tunnel: ["9011" ("CN") "2061" ("CN") "9012" ("CN")] -> w1072
        frame "返回请求应答", Default {
        }
        frame "上传数据" {
        }
        frame "返回执行结果" {
        }
      }
      n694 = local read "QN"() -> (w1071:string)
    }
    frame "剖面多参数S" {
      # "监测小时数据"
      n695 = global read "全局1.vi" "枚举"() -> (w1081:enum16{"返回请求应答", "上传数据", "返回执行结果"})
      n696 = case shown="\"上传数据\"" w1081 {
        tunnel: ["9011" ("CN") "2011" ("CN") "9012" ("CN")] -> w1080
        frame "返回请求应答", Default {
        }
        frame "上传数据" {
        }
        frame "返回执行结果" {
        }
      }
      n697 = local read "QN"() -> (w1079:string)
    }
    frame "提取小时数据" {
      # "监测小时数据"
      n698 = global read "全局1.vi" "枚举"() -> (w1090:enum16{"返回请求应答", "上传数据", "返回执行结果"})
      n699 = global read "断电保存全局.vi" "数据组合发送"() -> (w1087:bool)
      n700 = case shown="\"上传数据\"" w1090 {
        tunnel: ["9011" ("CN") "2061" ("CN") "9012" ("CN")] -> w1089
        frame "返回请求应答", Default {
        }
        frame "上传数据" {
        }
        frame "返回执行结果" {
        }
      }
      n701 = case shown="真" w1087 {
        tunnel: ["8" ("ST") "9" ("ST")] -> w1092
        frame False {
        }
        frame True {
        }
      }
      n702 = local read "QN"() -> (w1088:string)
    }
    frame "提取实时数据" {
      # "提取实时数据"
      n703 = global read "全局1.vi" "枚举"() -> (w1099:enum16{"返回请求应答", "上传数据", "返回执行结果"})
      n704 = case shown="\"上传数据\"" w1099 {
        tunnel: ["9011" ("CN") w1105 "9012" ("CN")] -> w1098
        frame "返回请求应答", Default {
        }
        frame "上传数据" {
          n705 = global read "全局 实时数据参数.vi" "实时数据参数"() -> (w1104:string)
          n706 = case shown="\"平行样测试\"" w1104 {
            tunnel: ["2011" ("CN") "2064" ("CN") "2063" ("CN") "2065" ("CN") "2066" ("CN") "fff" ("CN")] -> w1105
            frame "水样测试", Default {
            }
            frame "平行样测试" {
            }
            frame "加标回收测试" {
            }
            frame "空白测试" {
            }
            frame "跨度核查" {
            }
            frame "" {
            }
          }
        }
        frame "返回执行结果" {
        }
      }
      n707 = local read "QN"() -> (w1100:string)
    }
    frame "跨度核查" {
      # "跨度核查"
      n708 = global read "全局1.vi" "枚举"() -> (w1116:enum16{"返回请求应答", "上传数据", "返回执行结果"})
      n709 = case shown="\"上传数据\"" w1116 {
        tunnel: ["9011" ("CN") "2066" ("ST") "9012" ("CN")] -> w1115
        frame "返回请求应答", Default {
        }
        frame "上传数据" {
        }
        frame "返回执行结果" {
        }
      }
      n710 = local read "QN"() -> (w1113:string)
    }
    frame "提取加标回收" {
      # "提取加标回收"
      n711 = global read "全局1.vi" "枚举"() -> (w1124:enum16{"返回请求应答", "上传数据", "返回执行结果"})
      n712 = case shown="\"上传数据\"" w1124 {
        tunnel: ["9011" ("CN") "2063" ("ST") "9012" ("CN")] -> w1123
        frame "返回请求应答", Default {
        }
        frame "上传数据" {
        }
        frame "返回执行结果" {
        }
      }
      n713 = local read "QN"() -> (w1121:string)
    }
    frame "提取平行样" {
      # "提取平行样"
      n714 = global read "全局1.vi" "枚举"() -> (w1132:enum16{"返回请求应答", "上传数据", "返回执行结果"})
      n715 = case shown="\"上传数据\"" w1132 {
        tunnel: ["9011" ("CN") "2064" ("ST") "9012" ("CN")] -> w1131
        frame "返回请求应答", Default {
        }
        frame "上传数据" {
        }
        frame "返回执行结果" {
        }
      }
      n716 = local read "QN"() -> (w1129:string)
    }
    frame "空白测试", "零点核查" {
      # "零点核查"
      n717 = global read "全局1.vi" "枚举"() -> (w1140:enum16{"返回请求应答", "上传数据", "返回执行结果"})
      n718 = case shown="\"上传数据\"" w1140 {
        tunnel: ["9011" ("CN") "2065" ("ST") "9012" ("CN")] -> w1139
        frame "返回请求应答", Default {
        }
        frame "上传数据" {
        }
        frame "返回执行结果" {
        }
      }
      n719 = local read "QN"() -> (w1137:string)
    }
    frame "核查数据" {
      # "核查数据"
      n720 = global read "全局1.vi" "枚举"() -> (w1148:enum16{"返回请求应答", "上传数据", "返回执行结果"})
      n721 = case shown="\"上传数据\"" w1148 {
        tunnel: ["9011" ("CN") "2062" ("ST") "9012" ("CN")] -> w1147
        frame "返回请求应答", Default {
        }
        frame "上传数据" {
        }
        frame "返回执行结果" {
        }
      }
      n722 = local read "QN"() -> (w1145:string)
    }
    frame "提取集成干预" {
      # "核查数据"
      n723 = global read "全局1.vi" "枚举"() -> (w1156:enum16{"返回请求应答", "上传数据", "返回执行结果"})
      n724 = case shown="\"上传数据\"" w1156 {
        tunnel: ["9011" ("CN") "2082" ("ST") "9012" ("CN")] -> w1155
        frame "返回请求应答", Default {
        }
        frame "上传数据" {
        }
        frame "返回执行结果" {
        }
      }
      n725 = local read "QN"() -> (w1153:string)
    }
    frame "报警信息", "操作日志", "仪器参数" {
      n726 = global read "全局1.vi" "枚举"() -> (w1167:enum16{"返回请求应答", "上传数据", "返回执行结果"})
      n727 = case shown="\"上传数据\"" w1167 {
        tunnel: ["9011" ("CN") "3020" ("CN") "9012" ("CN")] -> w1166
        frame "返回请求应答", Default {
        }
        frame "上传数据" {
        }
        frame "返回执行结果" {
        }
      }
      n728 = Get Date/Time In Seconds() -> (seconds since 1Jan1904=w1164:timestamp)
      n729 = Format Date/Time String(time format string (%c)="%Y%m%d%H%M%S%3u" ("时间格式字符串(%c)"), seconds (now)=w1164) -> (date/time string=w1163:string)  [unwired: 1 in]
      n730 = Search and Replace String(input string=w1163, search string="." ("搜索字符串")) -> (result string=w1161:string)  [unwired: 6 in, 3 out]
    }
    frame "3090仪器参数" {
      n731 = global read "全局1.vi" "枚举"() -> (w1179:enum16{"返回请求应答", "上传数据", "返回执行结果"})
      n732 = case shown="\"上传数据\"" w1179 {
        tunnel: ["9011" ("CN") "3090" ("CN") "9012" ("CN")] -> w1178
        frame "返回请求应答", Default {
        }
        frame "上传数据" {
        }
        frame "返回执行结果" {
        }
      }
      n733 = Get Date/Time In Seconds() -> (seconds since 1Jan1904=w1176:timestamp)
      n734 = Format Date/Time String(time format string (%c)="%Y%m%d%H%M%S%3u" ("时间格式字符串(%c)"), seconds (now)=w1176) -> (date/time string=w1175:string)  [unwired: 1 in]
      n735 = Search and Replace String(input string=w1175, search string="." ("搜索字符串")) -> (result string=w1173:string)  [unwired: 6 in, 3 out]
    }
    frame "提取仪器参数" {
      n736 = global read "全局1.vi" "枚举"() -> (w1187:enum16{"返回请求应答", "上传数据", "返回执行结果"})
      n737 = case shown="\"上传数据\"" w1187 {
        tunnel: ["9011" ("CN") "3020" ("CN") "9012" ("CN")] -> w1186
        frame "返回请求应答", Default {
        }
        frame "上传数据" {
        }
        frame "返回执行结果" {
        }
      }
      n738 = local read "QN"() -> (w1185:string)
    }
    frame "系统状态" {
      n739 = local read "QN"() -> (w1193:string)
    }
    frame "运行模式" {
      n740 = local read "QN"() -> (w1197:string)
    }
    frame "测量周期" {
      n741 = local read "QN"() -> (w1201:string)
    }
    frame "超标留样" {
      n742 = local read "QN"() -> (w1205:string)
    }
  }
  n743 = Bundle By Name(cluster="数据块", "ST"=w21, "CN"=w24, "FLAG"=w23, "CP"=w2, "QN"=w14, "MN"="MN", "PW"="PW", "PNUM"=w15, "PNO"=w15) -> (w22:T1)
  n744 = call "HJ212-2017.vi"("PWD？"=FALSE, "数据段"=w22) -> ("通讯包字符串"=w28:string, "通讯包"=→"通讯包":T2)  [unwired: 7 in, 1 out]
  "通讯包字符串" <- w28
  n745 = String Length(string=w28) -> (length=→"长度":i32)
  "错误常量" <- "错误常量 2"
  "小时数据发送次数" <- 0 ("小时数据发送次数")
  "核查数据发送次数" <- 0 ("核查数据发送次数")
